vi "PECT - Scan_time gate - 2.vi"() -> ()   [LabVIEW 2012]
uses:
  <vilib>/DAQmx/read.llb/DAQmx Read (Analog 1D DBL 1Chan NSamp).vi
  <vilib>/DAQmx/read.llb/DAQmx Read (Analog Wfm 1Chan NSamp).vi
  <vilib>/DAQmx/write.llb/DAQmx Write (Analog Wfm 1Chan NSamp).vi
  <vilib>/Instr/_visa.llb/VISA Configure Serial Port (Instr).vi
  <vilib>/DAQmx/create/channels.llb/DAQmx Create Channel (AI-Voltage-Basic).vi
  <vilib>/DAQmx/configure/timing.llb/DAQmx Timing (Sample Clock).vi
  <vilib>/DAQmx/configure/task.llb/DAQmx Configure Logging (TDMS).vi
  <vilib>/DAQmx/configure/trigger.llb/DAQmx Start Trigger (Digital Edge).vi
  <vilib>/DAQmx/create/channels.llb/DAQmx Create Channel (AO-Voltage-Basic).vi
  <vilib>/DAQmx/miscellaneous.llb/DAQmx Fill In Error Info.vi
  Global_data.vi
  <vilib>/express/express analysis/Spectral/Block/exnSpectralBlock spectral measurements PSD poly.vi
  <vilib>/express/express analysis/Spectral/Block/exnSpectralBlock spectral measurements PSD WFM.vi
  <vilib>/express/express analysis/Spectral/XNode/ExpressSpectralMeasurementsBlockNode.xnode
  <resource>/objmgr/daqmx.rc
  <vilib>/measure/NI_MABase.lvlib
  <vilib>/Platform/NI_3dgraph.lvlib
  <vilib>/DAQmx/write.llb/DAQmx Write (Analog 1D Wfm NChan NSamp).vi
panel:
  in  "Open tdms":bool
  in  "Pulse generator":T1={"Waveform Type"=0, "Amplitude"=6.0, "Frequency"=1000.0} {"Frequency" format="%0.2p"; "Amplitude" format="%0.2p"; "Waveform Type" items=["Sine Wave", "Triangle Wave", "Square Wave", "Sawtooth Wave"]}
  out "Cur. X":dbl format="%#_4g"
  out "Old X":dbl
  out "Cur. Y":dbl format="%#_4g"
  out "Old.Y":dbl
  out "Compare X":dbl
  out "compareY":dbl
  out "y >= 0":bool
  out "x >= 0":bool
  out "move X":dbl
  out "move Y":dbl
  out "deltaY":dbl
  out "delta X":dbl
  in  "Move Distance":dbl=5.0
  in  "Emergency Stop":bool
  in  "Stop 3":bool
  in  "Home Y":bool
  in  "Home X":bool
  in  "Back":bool
  in  "Front":bool
  in  "Left":bool
  in  "Right":bool
  in  "Stop Scan":bool
  out "Start Pos. X":dbl=-22.5 format="%#.4f"
  out "Start. Pos.Y":dbl=18.8 format="%#.4f"
  out "열거형":T2(ring)
  out "숫자형":i32
  in  "Gate 2":dbl=50.0
  in  "Gate 1":dbl=25.0
  out "No.data":i32
  in  "Save Scan mode":bool caption="Save Process"
  in  "Plot style":i32(ring)=5 items=["cwLine"=1, "cwPoint"=2, "cwLinePoint"=3, "cwHiddenLine"=4, "cwSurface"=5, "cwSurfaceLine"=6, "cwSurfaceNormal"=7, "cwContourLine"=8, "cwSurfaceContour"=9]
  in  "Stop 4":bool
  in  "ViewMode":i32(ring) items=["cwViewXYPlane", "cwViewXZPlane", "cwViewYZPlane", "cwViewUserDefined"]
  in  "Scan":bool
  in  "Motor Trigger Source":tag="/Dev6/PFI1" caption="소스"
  in  "Open csv":bool
  in  "Tab Control 2":T3(tab)
  out "Hall sensors signal":waveform(dbl)[](graph)=[{"t0"=timestamp(3525645621.636764 s since 1904-01-01), "dt"=1.9999999999999944e-06, "Y"=array[2100 elements], "attributes"=variant("NI_ChannelName"=variant(string "Dev1/ai0"), "NI_UnitDescription"=variant(string "Volts"))}, {"t0"=timestamp(3525645621.636764 s since 1904-01-01), "dt"=1.9999999999999944e-06, "Y"=array[2100 elements], "attributes"=variant("NI_ChannelName"=variant(string "Dev1/ai0"), "NI_UnitDescription"=variant(string "Volts"))}]
  out "Feature Extraction":dbl(graph)=0.021153968958947764
  out "Waveform Graph 2":waveform(dbl)(graph)
  out "Power spectral density":cluster{"f0":dbl, "df":dbl, "magnitude":dbl[]}[](graph)=[{"f0"=0.0, "df"=238.09523809523876, "magnitude"=[-25.4340272409559, -28.495970805276507, -69.09064054555873, -79.11355871279994, -75.69366097931027, -84.18131507822396, -80.50168881348966, -82.72314293089615, -87.19630499623688, -82.83568021481967, -89.95290866002237, -85.90392585035596, -87.41269111550386, -91.40893948681482, -86.69370819914215, -93.36336146616782, -89.019380476413, -89.73232030153878, -94.58261196624535, -89.16287927388944, -94.965890302584, -91.86846413178648, -91.95327957161693, -97.62687167891286, -91.59993648735762, -97.30685711015555, -93.8350762480425, -93.27921214218685, -99.59438563802183, -93.1824258709588, -98.3113125531512, -95.45425138584356, -94.39327135467576, -100.65352961491782, -94.55889081970952, -99.40788907105079, -97.93617495318924, -96.19517579047603, -103.97036797797732, -96.40295202889732, -99.7036956909043, -99.48760137175819, -97.46192979187015, -106.29271483151813, -97.51447379981207, -99.86179280251669, -100.43811038443037, -97.59011642740829, -105.58363666166275, -99.01126121197593, -101.01575323613292, -101.90167607549864, -98.61952569586691, -106.73670466995647, -99.29976101634999, -101.54959604687718, -105.17330050767885, -100.09392305285375, -109.78264848704497, -100.98914236173123, -101.81665207962125, -105.42358374403365, -99.82880728595141, -107.07330885402075, -101.07712607444097, -101.03780825357597, -107.32811151840846, -101.221643458408, -105.63776326231454, -101.8420593566944, -101.80081629073969, -107.47915505307212, -101.12986632760553, -106.84901404755908, -102.73715610491038, -101.51552854007832, -107.28771371003282, -101.3928633472346, -107.44515355816633, -104.89304864643535, -103.1455098860718, -110.19910428997925, -102.73063833081197, -107.57101838377707, -104.90574568581201, -103.72599931018533, -109.97178587260123, -103.24611921258705, -108.36098023558972, -106.6408311450923, -104.73569536588386, -116.21683530762306, -105.02627439976544, -107.15856030450797, -109.81191038702062, -105.53476822084077, -119.10077766590356, -105.31867536160968, -106.9718410299748, -108.34458911268797, -104.70307996109247, -114.76704583683203, -106.29948298493936, -108.55077108437321, -112.16618350190343, -105.98453547558171, -114.68576835450673, -107.50968901677987, -107.89174277914348, -111.59875709602721, -106.69368240333122, -114.93273233954758, -105.23904516482949, -106.00272331017348, -110.36103151258544, -104.93177986717492, -110.8835476773746, -106.69346348818806, -106.66103973993782, -119.11729839814336, -108.06338160849775, -114.5879267769655, -108.59816838472844, -107.53189260743514, -114.07390818184973, -106.70996756049796, -113.27381274118753, -109.50270539577696, -107.37282420343303, -113.4779718725949, -106.04267666963091, -111.30294425571472, -112.46717993668915, -109.13164915488709, -116.65287200885172, -107.03002573045511, -110.21479040603631, -112.476075561056, -106.97710947409149, -119.42145279296255, -108.3200486628316, -110.46641858585929, -117.16650627564961, -109.73297826697552, -120.31689830731365, -107.19513745371916, -110.66663569403087, -113.30365980039964, -110.01971553524372, -123.68660617105166, -110.8171755739396, -111.11382172813546, -117.76239209582961, -109.49899370205401, -115.22252846498625, -111.1932077339224, -112.38235939086871, -118.22207022901702, -110.6546796895719, -116.97450780644367, -110.82401674194465, -111.96705198878843, -118.28092956599232, -110.5621503678909, -121.25720613496851, -111.98371482341479, -113.27928013246557, -111.96833712758355, -108.56859286664552, -120.32790468431601, -110.82699792221703, -110.79062667340345, -122.65756767769517, -110.48843456045427, -116.8782055296399, -115.43719816168479, -114.47619780315773, -121.42183196132746, -111.60631415727042, -120.68077308056417, -109.35478690141552, -109.03210709352732, -120.6260555904793, -109.47936424950136, -113.33719701518146, -112.88325992990137, -110.99901978536154, -123.19636626521421, -109.09861317900774, -113.33125158106256, -115.35673297389727, -112.77249677632989, -124.61163141716472, -114.68140920359865, -121.89642913325117, -115.47413298424323, -112.82196063671608, -127.87542521315149, -111.54178118788309, -113.6448752704395, -120.76569423868874, -112.98651214877823, -123.18868565400437, -115.41399838634062, -115.46853076016815, -116.40989072804102, -110.69611347288615, -132.23164080331392, -114.76376391429793, -121.7246597336247, -117.46893009589195, -114.01899156779395, -125.22079066032327, -114.59524199183258, -114.50034890537415, -122.9532092227648, -113.72727798159212, -125.65163915514907, -113.4793801211504, -110.4090756414644, -125.63592649005872, -114.22938378193007, -116.74947251106808, -121.60535557984142, -116.79385283402802, -122.44667696630361, -113.43873413563811, -123.28159708694415, -113.92892974938164, -114.01193823589753, -121.62751955742443, -118.76839573694522, -125.52998605097204, -115.19609643487229, -117.49409595176479, -117.08423885198002, -119.48314867245172, -125.01675515413412, -117.92668164142911, -115.55962389856793, -125.63488616674975, -119.11862859365166, -114.78860770332909, -117.18339781294443, -111.18063004722558, -118.31775966044624, -111.6867367949252, -114.57226159377, -119.36541212960576, -113.90245139442648, -132.46343443313128, -120.1282759002165, -121.05279009698619, -118.9115822659523, -121.23280439248342, -116.31914159559688, -127.38829313950257, -117.34673005740623, -115.95249861902771, -114.9301657394146, -123.22361802797445, -110.83274939062106, -116.16624248562111, -116.76753364192771, -113.94454545069023, -122.95736945775944, -118.66755800656253, -129.1462641201204, -116.6351050110328, -117.22529407303742, -123.80212197360244, -115.89792176423389, -114.25823938606595, -125.60467961977515, -114.59958849364433, -121.70071005514421, -118.25968972451209, -114.69929400946009, -123.88209034116528, -115.03869272537257, -117.52034211782204, -115.27990843516797, -117.85366603932033, -125.16865559622727, -118.21960424638507, -119.69008755413566, -117.24640963460672, -114.32867295013791, -119.1576982419508, -122.85495988425586, -116.3373010103401, -114.53730203699834, -115.67017599990201, -127.144321037601, -115.73849102686786, -117.7626163106355, -119.7346592991025, -117.41317517684553, -125.0417974461613, -114.5488949833583, -116.59812516173781, -119.91064563147799, -115.27933218667663, -122.09990513751134, -120.95678574143693, -123.25641714743752, -112.5173710452192, -113.53735878806998, -129.23914933506734, -116.27157269711533, -148.4020512032711, -118.84888216023774, -123.82550527215588, -116.87770979616658, -111.32191810025745, -124.32675905891588, -114.37182733794062, -121.10713785851372, -122.59698730059695, -116.38346694563282, -121.69144349152856, -119.00883142493832, -110.81886738196273, -120.7909830607913, -115.01780448665316, -114.52055121633796, -132.6824191654361, -116.330695115645, -126.4664151018508, -118.32717907779282, -118.7288071595281, -120.42749846140066, -112.53185615773879, -124.26026008984286, -114.24089252048742, -120.00368190003405, -114.71738500842926, -112.92262025927133, -129.21127897188563, -113.5947811765517, -117.80802009651353, -117.0133790103226, -112.19210322760304, -118.17549968071762, -119.3256187825503, -118.84981507334446, -121.39118969751144, -114.64543555194373, -119.84814933224528, -114.09123407848944, -116.22899352170892, -116.41650104077173, -113.70057202673476, -124.52773908304957, -114.87372641784933, -116.11651108221098, -121.68680962246994, -115.78306007961302, -122.22621008657796, -118.81157995182392, -113.9402115821658, -132.636729517989, -114.49554876936634, -119.50980190398928, -123.27410972236837, -118.52851881066383, -122.25212982572599, -117.13947036230024, -120.85005588797962, -118.41526503460501, -117.61788553858068, -126.3872056783977, -114.98198608543298, -119.7789938911847, -120.84873579392627, -114.38831474301695, -153.35954756825245, -113.19505610638078, -114.17454820985151, -127.41069917723112, -114.92677241657191, -125.49053973810628, -113.36382196587914, -119.96785250843519, -122.47388530423243, -116.38671253508838, -120.0905790211523, -119.83326265062107, -117.88168146696918, -122.3132169880757, -115.87324909105399, -125.92003267803432, -113.96860176867415, -114.49156118371398, -127.52634390035722, -115.05967156528004, -126.82020221981517, -117.93643187259194, -116.51163213641807, -119.47551219110167, -119.55225172256931, -116.9512257852571, -122.23153124485954, -120.8368476753637, -121.48473913072222, -115.83122660909913, -135.74260014140523, -116.58358375805423, -118.15236945484727, -119.06674062398864, -115.7844834762477, -125.06111738611818, -114.7801535050972, -115.2696605691888, -123.98656374010793, -119.29025555731172, -118.29146803784099, -119.55696172158135, -118.06884171238352, -127.81587648134607, -120.41730580797976, -123.49626136731604, -112.2147141798107, -116.22555232584983, -132.79419178871254, -119.66964883124663, -117.20946469243259, -118.20939292735417, -115.6951914646649, -129.64892855822356, -114.27056999288617, -120.31005512957381, -117.41846777372632, -115.50158386260813, -124.69777160737624, -115.2892897247205, -123.61522771666871, -113.75248734362687, -113.22999749252833, -129.3490509395313, -116.88137735661701, -116.94110280242681, -119.50244079984806, -119.30521139999144, -128.17199984115797, -118.06736594940236, -116.05331575995922, -121.29670750650897, -116.1140297602044, -125.090619084802, -121.41807296062154, -120.01332757902264, -120.54914530643151, -116.49738633175463, -122.32551291835904, -118.3190808346865, -118.92638453656723, -122.48819531011718, -117.01021725424317, -120.98896352560598, -117.23831688685218, -121.27915259197124, -121.20017251921661, -117.6155648860373, -120.91300272912063, -117.94438460863424, -115.94437430101533, -123.35904829443987, -117.74011174503076, -121.54935745388448, -120.82564553545025, -121.98951430455743, -120.24858103448778, -116.44403527138395, -112.79571494351876, -112.42801913096545, -110.1697573019791, -115.34500457736401, -119.81921052956707, -129.82600951154313, -115.5862301263047, -112.59292882433087, -120.79009137478283, -131.32849293387295, -113.61194478398238, -123.48568856527031, -119.17507777781304, -123.09261867490484, -116.97755217417308, -123.94453461434183, -116.58080525616379, -119.64289646280756, -122.90202645580743, -126.66219093058154, -121.95048829056148, -115.72578023509817, -116.70117814464484, -121.91050280869723, -118.25299095698178, -116.45905559047064, -132.57794493731578, -121.65327820443292, -120.9816664775787, -117.17270262269045, -120.27433984830965, -125.89418976028173, -119.09563505847817, -126.9693215534833, -113.17465524665704, -118.98702092883116, -119.83822568580342, -120.45832738089722, -120.67735960513633, -127.38676010839353, -127.65777338183055, -118.37446329057411, -115.61355494839711, -119.94568688114103, -116.06619937633681, -126.348857777089, -118.92850079147068, -119.5416617639739, -132.47075644221843, -118.08809356028496, -123.16186463092723, -121.51579486791232, -122.88983670053283, -129.5195538417256, -120.4730389608841, -132.16486858341602, -122.34690358436781, -120.71922104337597, -114.29260860841114, -117.67902631803368, -124.7040155514909, -123.51274592117205, -120.02297921674332, -136.54655493811157, -120.45629227407751, -119.06410204276258, -127.91681714792554, -122.82090055753153, -125.16838176650813, -121.79565386970478, -119.79607311590995, -126.54861375039647, -121.59135878113302, -132.8348640697562, -118.1305434733294, -120.46070148841905, -122.69571910896963, -117.6534954653865, -124.15742546824006, -120.73646926947502, -124.82696993800742, -124.513836786494, -123.15395713389651, -124.62395468806395, -117.21365768658171, -119.32635871968456, -121.48532284413152, -119.38242892643675, -126.25575652510352, -123.27133124029851, -117.58533922728374, -118.17710108929799, -114.99496360200965, -117.77133194647278, -111.34898201101595, -111.50817058307922, -119.0703124690998, -127.70676079885351, -121.8704969141074, -125.93154214283446, -118.65628450081473, -122.47918878348962, -117.9651589546518, -126.13560583004508, -122.42294805637847, -133.924453763793, -117.2082573038767, -117.6525335446734, -122.92077297426977, -122.04624645756786, -116.43289028226238, -117.93180959338378, -129.02356734231915, -117.95493621286326, -120.7555929766252, -120.76782849311112, -123.06287498470708, -117.83798593857965, -123.43423215434719, -120.15190119516652, -120.48240443128407, -143.29738987393452, -123.46572247444769, -120.89055325172792, -125.66715973809033, -118.26887578998644, -117.01836200028421, -121.33021830755509, -119.68846363313813, -122.60689066103069, -116.26858138914181, -119.59360791972998, -122.94866175463353, -114.174409515556, -118.00516930888391, -121.56978543579633, -135.87799017759036, -117.50816594504829, -122.82539428457626, -123.82103443155845, -124.77975840345442, -121.13340798086698, -120.93607435603558, -133.15787160745222, -120.70545628137863, -125.02155972441679, -122.04666465472178, -118.01234649746348, -127.88767491042842, -119.02096620167217, -120.16031065152875, -122.25406107859625, -121.72733059051095, -120.61357375519918, -118.63962847172827, -134.3857741605498, -116.3600853185034, -117.26695700691671, -119.9176982185873, -113.45576465218444, -126.69779573632724, -114.39554522802246, -116.8457146515868, -116.34219889483086, -119.30011291548334, -120.01163291843496, -114.29497178248809, -127.65687642749229, -119.58556923753022, -129.8593054181261, -122.2353645100479, -120.79536520223796, -119.83284028355028, -117.7991246185715, -128.390292904734, -119.78079925213122, -125.478913448993, -113.89747777944768, -112.66620124153357, -124.3475049842711, -120.85847303094337, -132.91807981902295, -119.523494985723, -116.65149909866443, -119.73287290436721, -127.63237851524192, -127.23413304048789, -120.87585453904362, -121.08540368080186, -134.91071939669257, -117.75375801669338, -117.2683014590723, -120.9739099492833, -118.23809733632451, -120.94065804928206, -123.88077510875804, -118.13812819300607, -122.60294123365466, -126.97075898006995, -120.18754789731035, -124.71238663441227, -120.55456557278582, -130.94599087480253, -111.18288669417035, -112.27708791831247, -126.0512034600378, -117.41881712783596, -128.20553880273903, -117.29482600885808, -118.2045526390752, -127.81966672699878, -117.03716165902529, -115.46711739757512, -117.15363929234843, -121.87599671671335, -121.19736800869221, -126.5301786755875, -131.20754947382918, -124.40138004810741, -129.0562496906515, -121.06816554587536, -121.01023627802867, -138.6137911215848, -120.12495002524031, -121.38510517514229, -122.79804220535513, -116.97501378195477, -118.82011581137473, -114.0229185604644, -119.54287501990726, -114.64474566771625, -117.76935669872461, -123.81082574158907, -118.51678358865587, -128.9664755188374, -123.45357998434133, -122.74888841574231, -120.74640581234044, -126.956344345126, -119.95682140104577, -118.8873101779055, -124.41062359284174, -128.97304498664363, -123.86287113204068, -127.30257087528216, -120.61364220528216, -114.45119129304715, -119.68384044686806, -131.29639185291157, -122.31250766293485, -119.57420865241102, -124.74014026002448, -124.87593035709094, -118.4566565612952, -123.76236085976001, -120.84780538841838, -117.68987599773281, -135.06195695255914, -122.56143585795171, -129.04610316842883, -118.32313199570537, -117.77093802786419, -124.46572845786741, -129.1123298336903, -120.88470269965448, -116.69988985752187, -116.84054667499878, -133.76883696987278, -122.32434984927302, -124.98940594457933, -122.56515592789917, -118.31562562243366, -133.97049179545627, -122.33220627999802, -131.16753675316977, -124.69828063969263, -116.37621154460467, -126.1833423168025, -129.62937634161355, -118.46241371150788, -117.52851478852457, -125.32425037236442, -119.0327364293772, -124.2861355894013, -123.24573502278234, -125.52155812053758, -113.75743410709823, -114.79513162658353, -128.58142362588052, -122.48277095196701, -118.94747544412269, -123.86988127835491, -124.78140456983323, -121.53998481875398, -116.01432822539552, -119.20174681160661, -122.75167725800814, -120.58657749420254, -118.51141061842183, -119.24457006171983, -131.43641234223372, -116.00759139055087, -121.24442216102587, -123.29371279953725, -117.608355420454, -116.33684374617326, -118.06291688281922, -121.88761866022774, -121.54820313120047, -119.5051369873635, -126.56611158390913, -118.84012713615805, -121.09285296522563, -124.67955377692547, -147.31451139022337, -116.80660421066897, -114.8367853755961, -120.41026468628925, -123.65666101895222, -119.64837119787269, -116.77480172559095, -116.54263359173909, -124.75286620868079, -117.33721912698883, -116.51795620907136, -118.50086748176733, -128.10381328920522, -122.78098994574157, -120.24716756092855, -119.52743204722819, -115.00407387659232, -108.2853711552629, -108.61086943894702, -119.6228894146785, -124.11132022420912, -125.6202218409766, -123.1749360787656, -118.1971196161698, -123.95075368058998, -121.72140109898365, -123.27106899042522, -123.73035629887062, -121.24369679109273, -121.07381526465288, -113.13965659723667, -118.330755475899, -118.40249076804484, -111.59630598649044, -116.1569506845575, -125.67326089915758, -125.85723567111906, -119.24293277595024, -117.87067617433537, -120.70936924059559, -131.8090588468898, -132.98711569625004, -123.63274249467587, -122.75476917502559, -126.12873814250243, -120.53144270605179, -129.07030822919336, -122.7889410422919, -124.35405971166259, -119.63968579420454, -139.0154441054289, -129.47962001806934, -121.86548015410847, -128.6818469257012, -121.40195873232601, -138.64231053781285, -124.22025721762265, -124.06073958736941, -126.71929802352521, -131.7498459276443, -120.68144109742178, -122.6325588818875, -126.80796617875095, -124.92487955227033, -136.94498040498806, -124.26704334219014, -123.21376211221711, -140.25352033075964, -129.53222319772195, -122.58541579060463, -122.1996729592375, -125.66642108013673, -125.66310429236694, -120.09682773706965, -125.27326633941439, -121.55721878725502, -121.22507119941083, -121.53716878624485, -136.20685498111987, -128.15260146013156, -120.03473972471616, -124.60755958763912, -124.73082500077143, -123.93425949983688, -131.04483249265184, -121.7957035014449, -127.09321441816094, -133.6144579272493, -124.69014595896968, -130.4902091211609, -121.18031440773905, -128.00033943961677, -125.88991118115149, -118.865310745079, -123.69668867733147, -117.98756965862728, -114.40013091842827, -118.28685032521078, -122.23464196869948, -124.8440422629961, -129.66281606870848, -119.440534215621, -124.54391783563877, -124.93447967158188, -121.7258558761523, -122.28817885403082, -127.06889620458577, -128.92172974939206, -120.62932166634072, -126.06847321900452, -123.31471168429935, -121.80350826545656, -129.2574604322076, -125.67225933193998, -125.7801671825605, -129.53804733161627, -119.56756644124712, -128.82490314699373, -124.7689736295626, -120.50019729114693, -124.50603158563972, -122.8120627011088, -125.60528875555717, -123.8817354922713, -124.05570537836674, -120.94568834491936, -118.06056028605255, -124.24390361274648, -125.5716703018188, -127.71949519914061, -130.7001652968252, -126.27701412017494, -133.76810134709916, -128.4738939614179, -120.302550881701, -118.91298143662928, -124.9077318110765, -127.16253699189492, -118.11405934812818, -117.52028071290711, -140.95620572748925, -123.61977932545628, -131.0334379970501, -125.88948384968432, -127.81552331993379, -121.92316280719056, -119.05911238768732, -126.83773251459189, -123.52627415002164, -120.8779561023192, -123.66683567603742, -131.64300993967345, -123.62895847772963, -116.89792951363142, -120.1068259250195, -117.92484706459337, -115.58208487778379, -120.76803581628594, -123.95408562090736, -122.79456549632754, -134.5305398779298, -123.57040300991032, -128.40634159414552, -123.70102187824159, -118.24970739397313, -119.66483900349026, -127.78024313111393, -120.3547204111785, -125.49305364308705, -119.49505591004302, -120.50920386196539, -119.03509516851003, -114.24667300009652, -121.60538636584391, -119.95304417598024, -122.24585853682832, -128.63653016912684, -116.04810628805795, -121.94159862131235, -122.59928204398939, -121.4532410501923, -128.6511474663462, -130.83715595958148, -121.71998300574741, -116.91426629511156, -113.587592058512, -115.59736707638731, -124.65300822631244, -133.32538684258748, -124.02289142873636, -121.54278890993639, -119.02596809402394, -108.90572887117857, -112.14974069608851, -129.21149299565423, -118.82148342951197, -116.65510894288538, -118.39609618084175, -116.53502642884725, -122.47549439965209, -122.23125657046063, -123.68081343116663, -120.67915071600007, -123.6899360128769, -118.56721985209728, -118.36641581191942, -126.96724630704657, -119.36877661672403, -123.07698921198843, -117.80772421906035, -122.82545076270567, -118.82755071380888, -117.21030132539394, -129.760567864525, -118.0816708063509, -125.80573274113647, -121.18434666182338, -121.80987210832065, -130.99259828357094, -125.47223579895922, -123.86818606677002, -118.7118158196511, -119.27778317338742, -127.27333258839096, -119.90672352079164, -140.78772370844268, -118.08251080057329, -119.86636232122572, -118.69482489738232, -119.19106512767372, -123.70988914879189, -121.92566832147995, -123.41378261726373, -120.1715186070818, -117.9079629421116, -117.41960207545632, -123.72833996166874, -127.24377206607298, -124.99098647980887, -129.48803701799955, -129.92351350561592, -120.79284154834647, -119.29601975194524, -136.17244775530037, -126.73975437546255, -128.84068276143336, -125.66374985701982, -136.69026010435715, -125.44409235146617, -119.28138070315057, -118.65017329869724, -118.02521532826772, -122.23736063759657, -121.27846943548622, -116.69850478126861, -119.7711336696722, -123.70776561180185, -118.43344549561263, -123.92390877157247, -117.19637143066551, -117.64112988205311, -127.78399195238529]}, ...(2 in all)]
  in  "3D Surface":refnum<k7>(container)
  out "Record path":path caption="selected path"
  out "Feature Extraction 2":dbl(graph)=0.021153968958947764
  in  "Tab Control":T4(tab)
  in  "Step X":dbl=0.1
  out "Move X":bool
  in  "Direction (+)":bool=TRUE
  in  "Step Y":dbl=0.1
  in  "Y-length":dbl=10.0
  in  "X-length":dbl=5.0
  in  "Save Speed":bool
  in  "Cur. Pos Y":dbl=18.8 format="%#.4f"
  in  "Cur. Pos X":dbl=-22.5 format="%#.4f"
  in  "Travel per Pulse (mm)":dbl=0.002
  in  "2 Rate":dbl=0.2
  in  "1 Rate":dbl=0.2
  in  "2 Min":dbl=1.0
  in  "1  Max":dbl=8.0
  in  "2 Max":dbl=8.0
  in  "1 Min":dbl=1.0
  in  "Parity":u16(ring) items=["None", "Odd", "Even", "Mark", "Space"]
  in  "stop bits":u16(ring)=10 items=["1.0"=10, "1.5"=15, "2.0"=20]
  in  "Data bits":u16=8 min=5 max=8 step=1
  in  "Baud Rate":u32=9600
  in  "COM Port":refnum<visa-resource-name>="COM12"
  out "No. X":i32
  out "No. Y":i32
  out "Sample per Channel AI":dbl
  out "Sample per Channel AO":dbl
  in  "Pulser Cycles":i32=10
  in  "Logging Mode":i32(ring)=10231 items=["Off"=10231, "Log and Read"=15842]
  out "Actual Sample Rate":dbl=500000.0 format="%0.2f"
  in  "Physical Channel":tag="Dev6/ai0"
  in  "Min Voltage":dbl=-10.0
  in  "Max Voltage":dbl=10.0
  in  "Terminal Configuration":i32(ring)=10083 items=["default"=-1, "RSE"=10083, "NRSE"=10078, "Differential"=10106, "Pseudodifferential"=12529]
  in  "Sample Clock Source 2":tag="OnboardClock"
  in  "Sample Rate":dbl=500000.0
  in  "TDMS File Path":path
  out "Actual Sample Rate 2":dbl=800000.0 format="%0.2f"
  in  "Physical Channel(s)":tag="Dev6/ao1"
  in  "Min Voltage 2":dbl=-10.0
  in  "Max Voltage 2":dbl=10.0
  in  "Sample Clock Source":tag="OnboardClock"
  in  "Sample Rate 2":dbl=800000.0
  in  "Offset":bool
  in  "2 Plots":bool
  in  "Edge":i32(ring)=10280 items=["Rising"=10280, "Falling"=10171]
  in  "Pulser Trigger Source":tag="/Dev6/PFI0"
  in  "Duty cycle %":dbl=50.0 format="%#.2f"
  # "Pulse Shape"
  # "Trigger Settings"
  # "Data Processing"
  # "Time gate = %T"
  # "Pulse"
  # "Hall Sensors Signal"
  # "Feature Extraction"
  # "Power Spectal Density"
  # "COM  Setting"
  # "Speed  Setting"
  # "Scan  Setting"
  # "Pulse  Channel"
  # "Pulse  Timming"
  # "Sensor  Channel"
  # "DAQ Timming"
  # "Logging Settings"
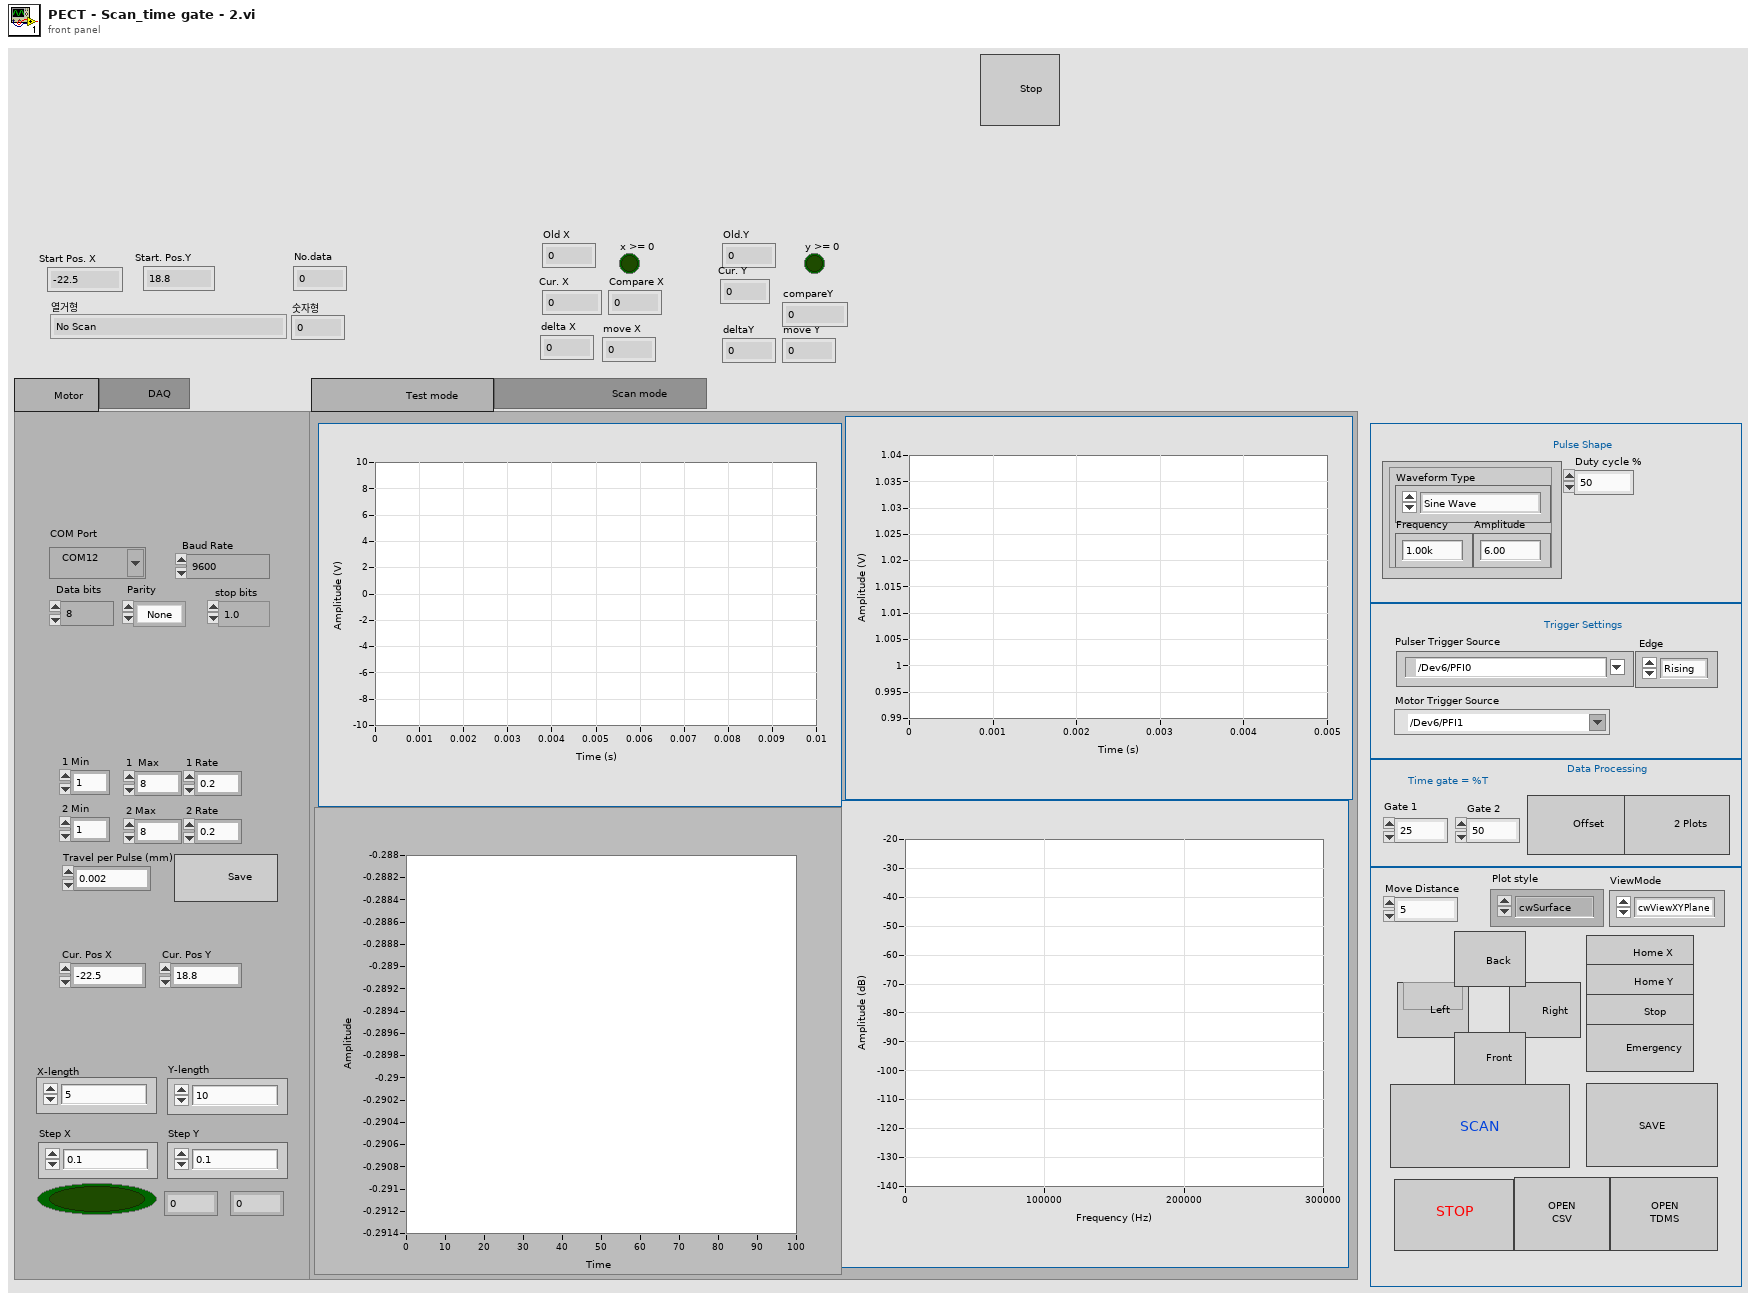
[diagram p1: front panel]
types:
  T1 = cluster{"Waveform Type":u16, "Amplitude":dbl, "Frequency":dbl}
  T2 = enum16{"No Scan", "Move X", "Wait to destination X", "Move Y", "Wait to destinatioin Y"}
  T3 = enum32{"                    Test mode                   ", "                          Scan mode                      "}
  T4 = enum32{"        Motor      ", "          DAQ        "}
  T5 = enum16{"open", "open or create", "create or replace", "create", "open (read-only)"}
  T6 = cluster{"averaging mode":u16, "weighting mode":u16, "number of averages":u32}
  T7 = cluster{"dB On (F)":bool, "unwrap phase (F)":bool, "convert to degree (F)":bool}
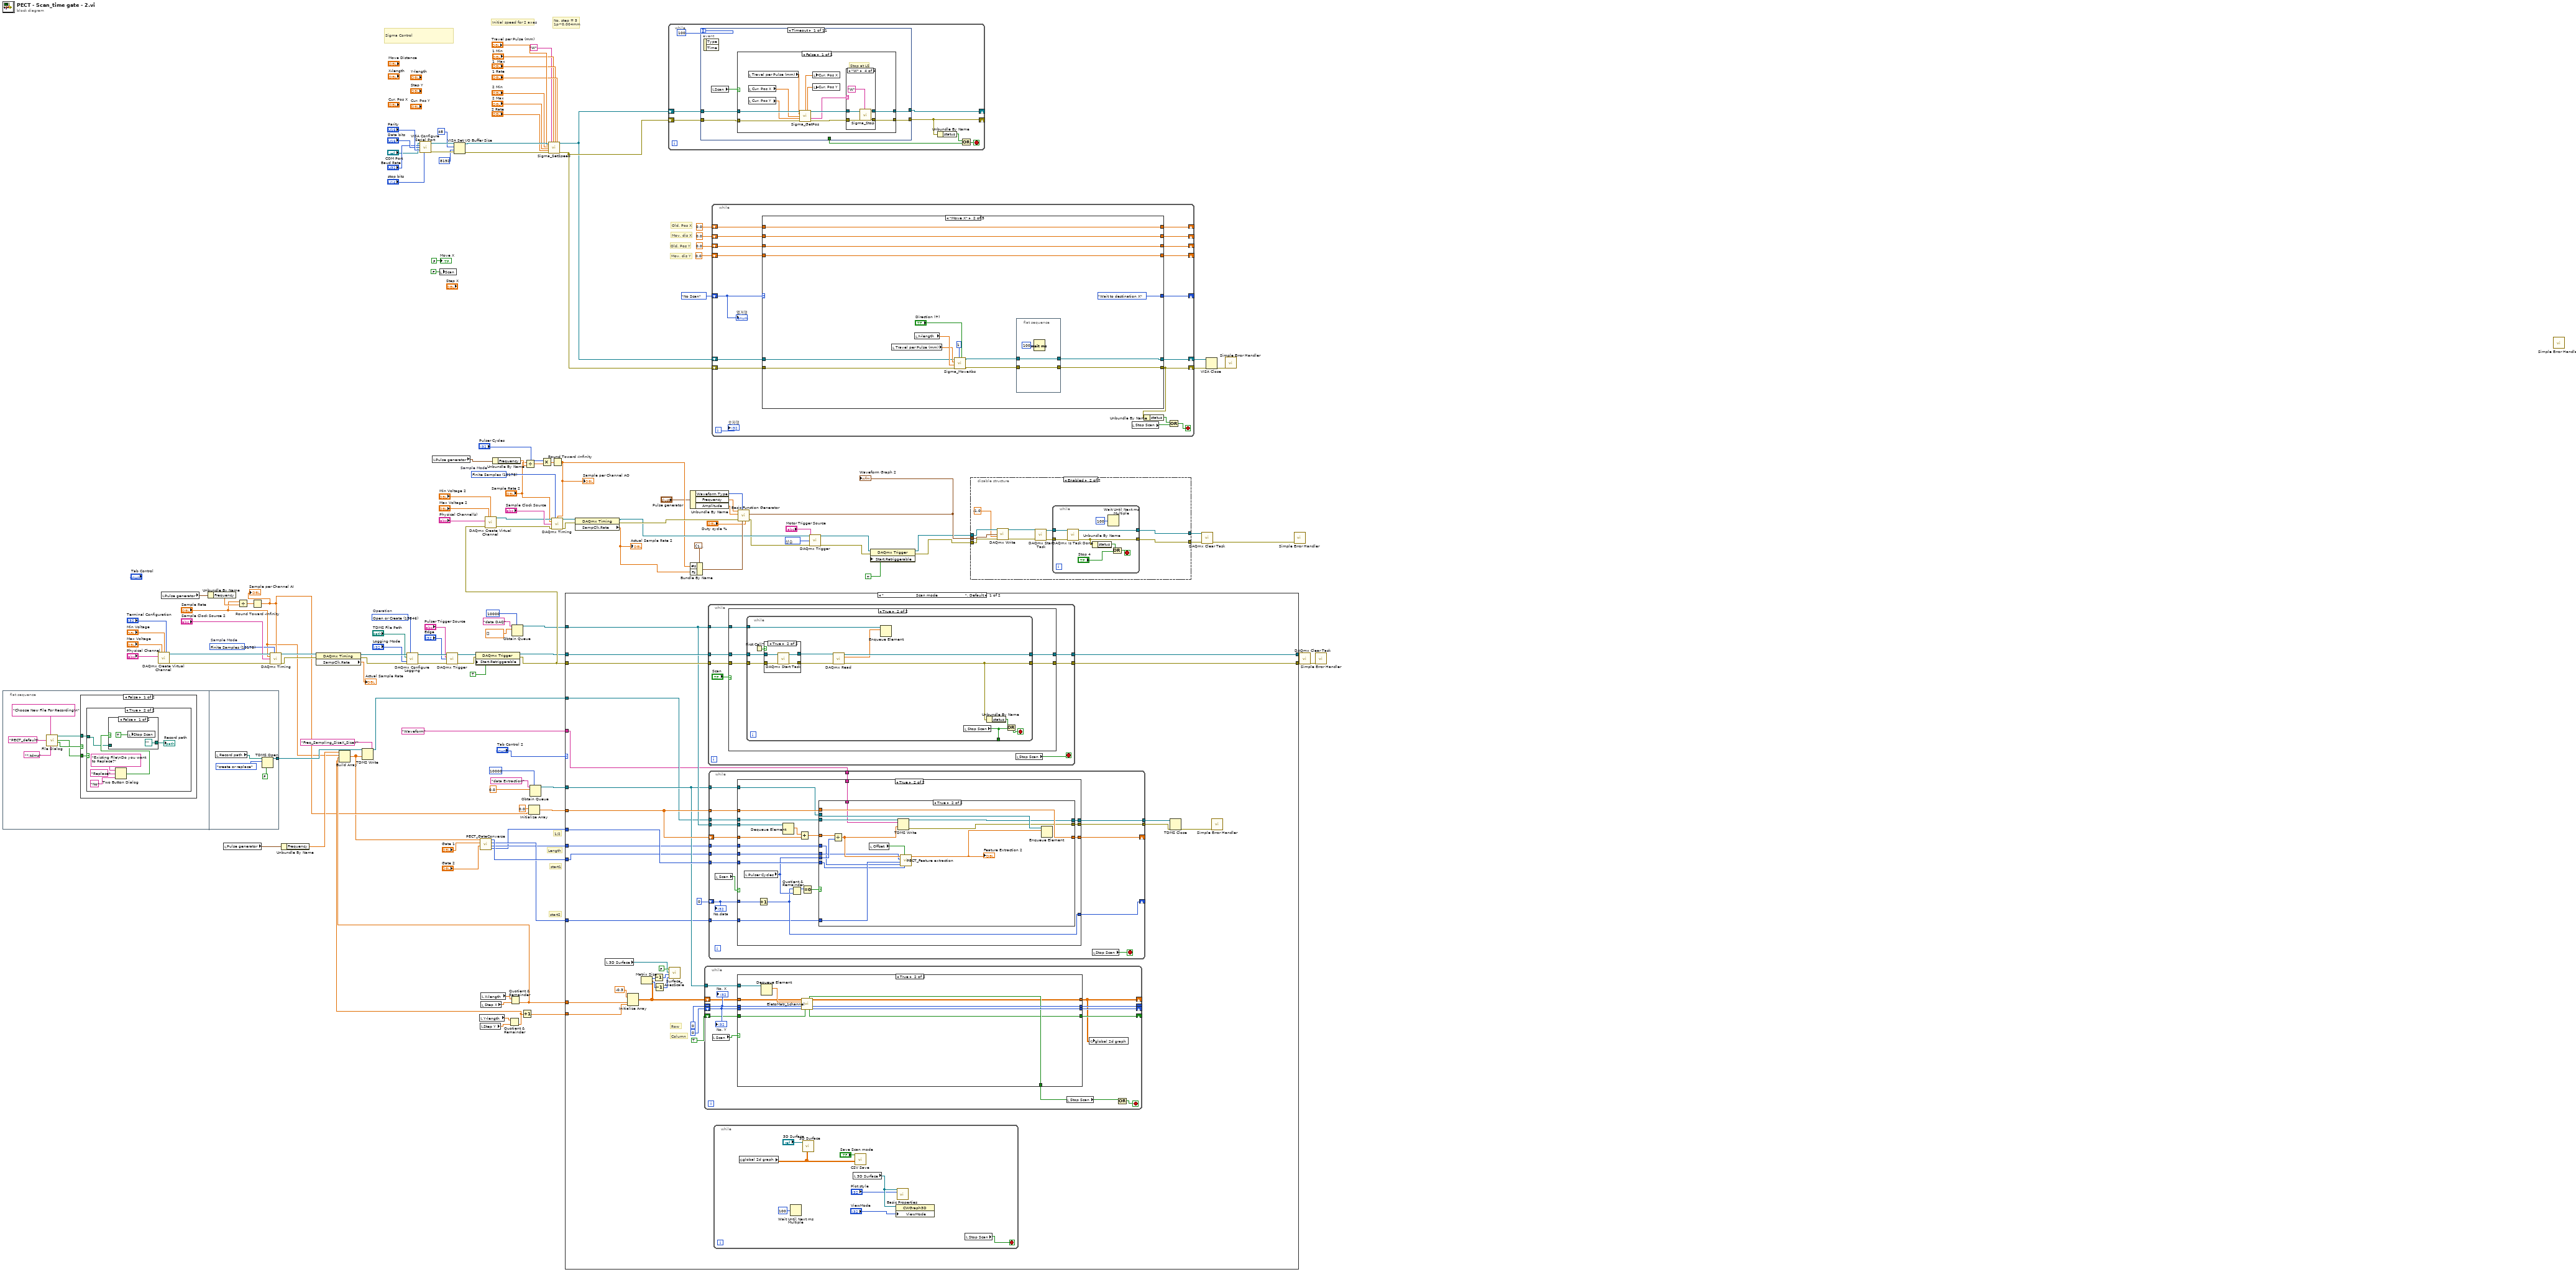
[diagram p0: block diagram]
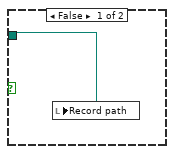
[diagram p2: hidden frame]
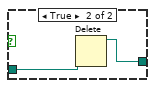
[diagram p3: hidden frame]
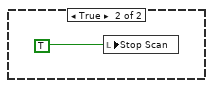
[diagram p4: hidden frame]
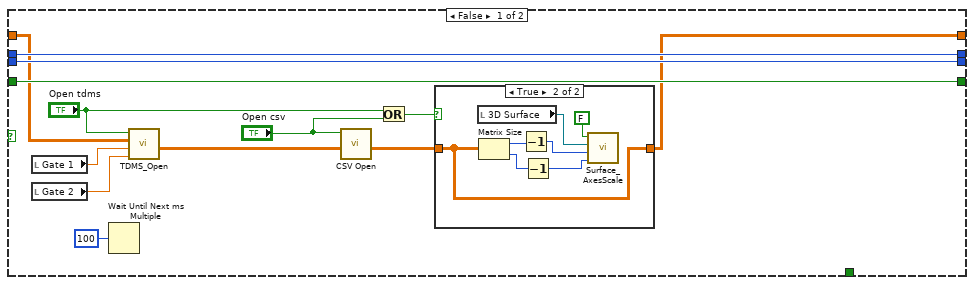
[diagram p5: hidden frame]
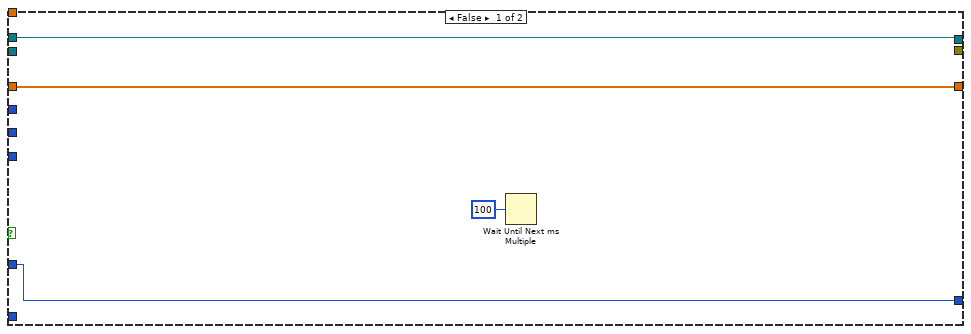
[diagram p9: hidden frame]
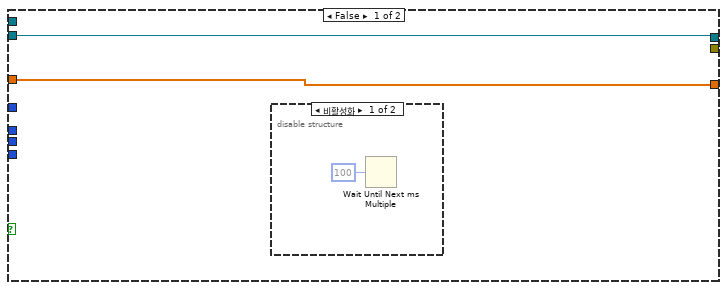
[diagram p10: hidden frame]
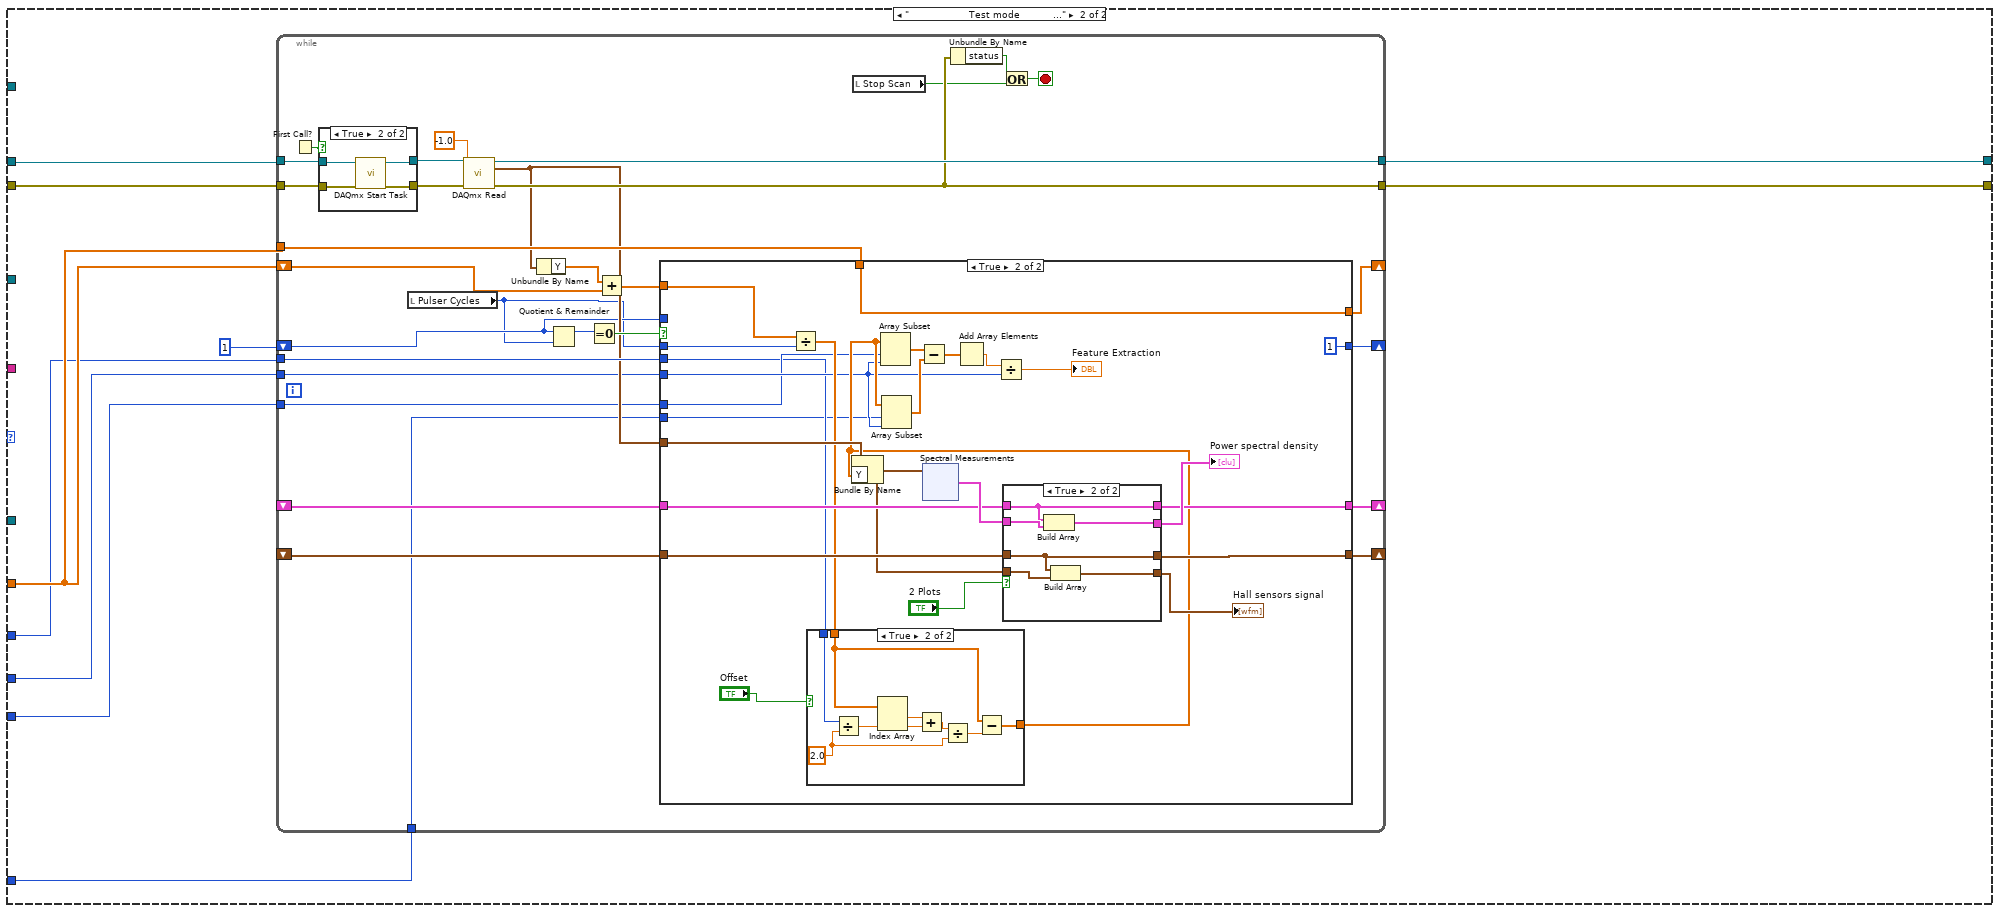
[diagram p12: hidden frame]
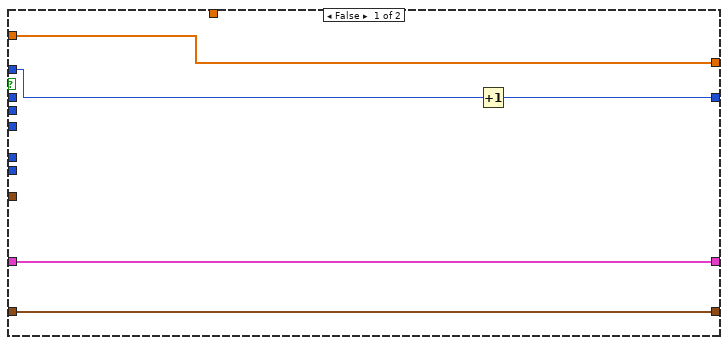
[diagram p14: hidden frame]
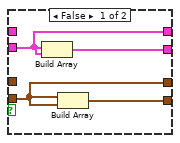
[diagram p16: hidden frame]
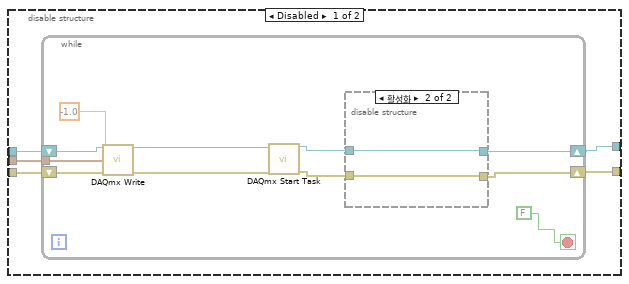
[diagram p17: hidden frame]
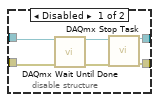
[diagram p18: hidden frame]
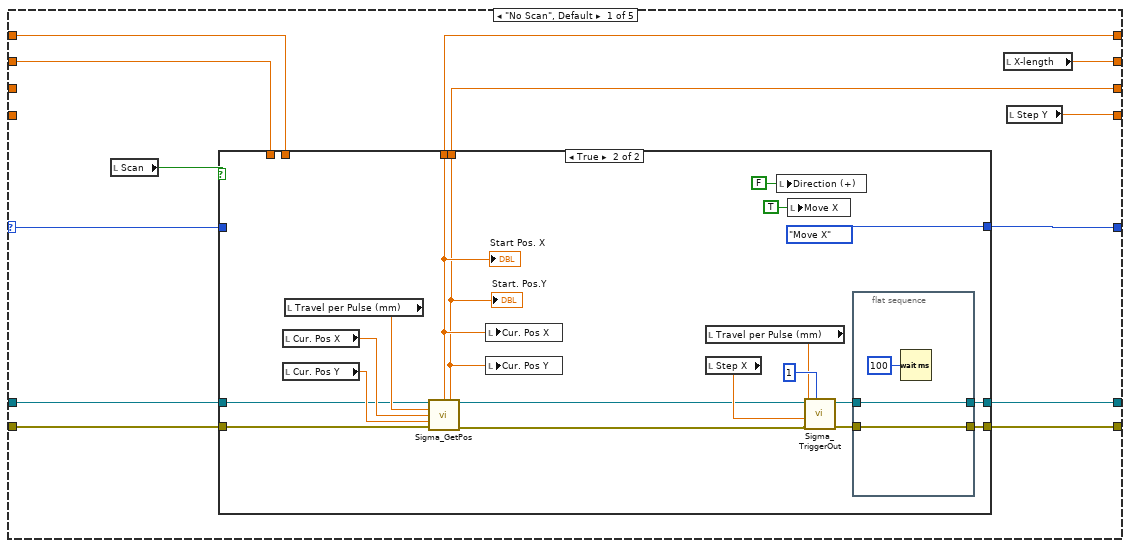
[diagram p19: hidden frame]
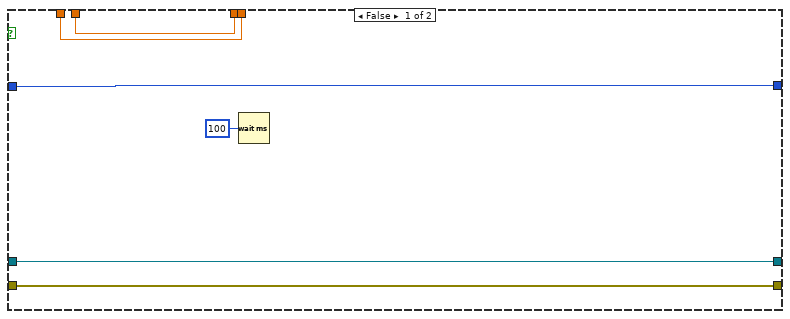
[diagram p20: hidden frame]
diagram:
  w51 = 10178 items=["Finite Samples"=10178, "Continuous Samples"=10123, "Hardware Timed Single Point"=12522]  # Sample Mode
  w66 = 15846 items=["Open"=10437, "Open or Create"=15846, "Create or Replace"=15847, "Create"=15848]  # Operation
  w89 = 10280 items=["상승"=10280, "하강"=10171] ("edge")
  w103 = 10178 items=["Finite Samples"=10178, "Continuous Samples"=10123, "Hardware Timed Single Point"=12522]  # Sample Mode
  # "1/2"
  # "start1"
  # "start2"
  # "Length"
  # "Mov. dis Y"
  # "Old. Pos Y"
  # "Mov. dis X"
  # "Old. Pos X"
  # "No. step = 5\n1p~0.004mm"
  # "Initial speed for 2 axes"
  # "Sigma Control"
  n1 = flat-sequence {
    tunnel: [w155] -> w27
    frame #0 {
      n2 = call "File Dialog"("prompt"="Choose New File For Recording\n" ("button label"), "default name"="PECT_default", "pattern (all files)"="*.tdms") -> ("selected path"=w139:path, "exists"=w134:bool, "cancelled"=w135:bool)  [unwired: 9 in, 1 out]
      n3 = case shown="False" w135 {
        tunnel: w139 -> [w140 _]
        tunnel: w134 -> [w141 _]
        frame False {
          n4 = case shown="True" w141 {
            tunnel: w140 -> [w142 w143]
            frame False {
              n5 = local write "Record path"(w142) -> ()
            }
            frame True {
              n6 = Two Button Dialog(message="Existing File\nDo you want to Replace?", 1:"No" ("F button name (\"Cancel\")"), 2:"Replace" ("T button name (\"OK\")")) -> (T button?=w144:bool)
              n7 = case shown="False" w144 {
                tunnel: w143 -> [_ w152]
                tunnel: [path "" ("deleted path") w151] -> w145
                frame False {
                  n8 = local write "Stop Scan"(TRUE ("Exit")) -> ()
                }
                frame True {
                  n9 = Delete(path (use dialog)=w152) -> (deleted path=w151:path)  [unwired: 4 in, 2 out]
                }
              }
              "Record path" <- w145
            }
          }
        }
        frame True {
          n10 = local write "Stop Scan"(TRUE ("Exit")) -> ()
        }
      }
    }
    frame #1 {
      n11 = local read "Record path"() -> (w154:path)
      n12 = TDMS Open(6:FALSE ("disable buffering (T)"), 10:T5."create or replace" ("operation"), 11:w154) -> (3:w155:refnum<k34>)  [unwired: 3 in, 1 out]
    }
  }
  n13 = call-poly <vilib>:"DAQmx Create Virtual Channel.vi"("maximum value"="Max Voltage", "minimum value"="Min Voltage", "input terminal configuration"="Terminal Configuration", "physical channels"="Physical Channel") -> ("task out"=w69:refnum<k21>, "error out"=w70:errorcluster)  [unwired: 10 in]
  n14 = local read "Pulse generator"() -> (w3:T1)
  n15 = Unbundle By Name(w3) -> ("Frequency"=w31:dbl)
  n16 = local read "Pulse generator"() -> (w2:T1)
  n17 = Divide(x="Sample Rate", y=w31) -> (x/y=w30:dbl)
  n18 = Round Toward -Infinity(1:w30) -> (0:w20:dbl)
  "Sample per Channel AI" <- w20
  n19 = call-poly <vilib>:"DAQmx Timing.vi"("task/channels in"=w69, "sample mode"=w51, "samples per channel"=w20, "rate"="Sample Rate", "source"="Sample Clock Source 2", "error in"=w70) -> ("task out"=w72:refnum<k21>, "error out"=w71:errorcluster)  [unwired: 8 in]
  n20 = Unbundle By Name(w2) -> ("Frequency"=w21:dbl)
  n21 = property class="DAQmx Timing"(reference=w72, error in=w71) -> (reference out=w68:refnum<k21>, error out=w67:errorcluster, "SampClk.Rate"=→"Actual Sample Rate":dbl)
  n22 = call-poly <vilib>:"DAQmx Configure Logging.vi"("task/channels in"=w68, "operation"=w66, "file path"="TDMS File Path", "logging mode"="Logging Mode", "error in"=w67) -> ("task out"=w65:refnum<k21>, "error out"=w64:errorcluster)  [unwired: 9 in]
  n23 = call-poly "VISA Configure Serial Port"("VISA resource name"="COM Port", "baud rate (9600)"="Baud Rate", "data bits (8)"="Data bits", "parity (0:none)"="Parity", "stop bits (10: 1 bit)"="stop bits") -> ("VISA resource name out"=w120:refnum<visa-resource-name>, "error out"=w126:errorcluster)  [unwired: 9 in]
  n24 = local read "Pulse generator"() -> (w1:T1)
  n25 = local write "Scan"(FALSE ("Scan")) -> ()
  n26 = call-poly <vilib>:"DAQmx Trigger.vi"("task/channels in"=w65, "source"="Pulser Trigger Source", "edge"="Edge", "error in"=w64) -> ("task out"=w48:refnum<k21>, "error out"=w47:errorcluster)  [unwired: 10 in]
  n27 = VISA Set I/O Buffer Size(VISA resource name=w120, mask (16)=48, size (4096)=u32 8192, error in (no error)=w126) -> (VISA resource name out=w116:refnum<visa-resource-name>, error out=w117:errorcluster)
  n28 = property class="DAQmx Trigger"(reference=w48, error in=w47, "Start.Retriggerable"=TRUE) -> (reference out=w29:refnum<k21>, error out=w73:errorcluster)
  n29 = local read "Y-length"() -> (w35:dbl)
  n30 = local read "Step Y"() -> (w36:dbl)
  n31 = local read "X-length"() -> (w38:dbl)
  n32 = local read "Step X"() -> (w37:dbl)
  n33 = call-poly <vilib>:"DAQmx Create Virtual Channel.vi"("maximum value"="Max Voltage 2", "minimum value"="Min Voltage 2", "physical channels"="Physical Channel(s)", "error in"=w73) -> ("task out"=w88:refnum<k21>, "error out"=w87:errorcluster)  [unwired: 10 in]
  n34 = Unbundle By Name(w1) -> ("Frequency"=w79:dbl)
  n35 = Quotient & Remainder(x=w35, y=w36) -> (floor(x/y)=w23:dbl)  [unwired: 1 out]
  n36 = Quotient & Remainder(x=w38, y=w37) -> (floor(x/y)=w25:dbl)  [unwired: 1 out]
  n37 = Build Array(w21, "Sample Rate", w25, w23) -> (w15:dbl[])
  n38 = TDMS Write(0:w27, 5:"Freq_Sampling_SizeX_SizeY" ("group name in (Untitled)"), 9:w15) -> (4:w26:refnum<k34>)  [unwired: 3 in, 3 out]
  n39 = call "PECT_GateConverse.vi"("Gate 2"="Gate 2", "Gate 1"="Gate 1", "Freq_Sampling_SizeX_SizeY"=w15) -> ("Length T/2"=w9:i32, "Length"=w10:i32, "Start 2"=w11:i32, "Start 1"=w12:i32)  [unwired: 5 in]
  n40 = Obtain Queue(max queue size (-1, unlimited)=10000, name (unnamed)="data DAQ", element data type=dbl[] [] ("data")) -> (queue out=w43:refnum<queue>)  [unwired: 2 in, 2 out]
  n41 = Increment(x=w23) -> (x+1=w24:dbl)
  n42 = Divide(x="Sample Rate 2", y=w79) -> (x/y=w77:dbl)
  n43 = Initialize Array(0.0 ("element"), w20) -> (w44:dbl[])
  n44 = Obtain Queue(max queue size (-1, unlimited)=10000, name (unnamed)="data Extraction", element data type=0.0) -> (queue out=w41:refnum<queue>)  [unwired: 2 in, 2 out]
  n45 = Multiply(x="Pulser Cycles", y=w77) -> (x*y=w75:dbl)
  n46 = call "Sigma_SetSpeed.vi"("VISA resource name"=w116, "Travel per Pulse (0.004mm)"="Travel per Pulse (mm)", "Min (1mm) 2"="2 Min", "Max (2mm) 2"="2 Max", "Rate (1mm) 2"="2 Rate", "error in (no error)"=w117, "Axis (1)"="W", "Min (1mm)"="1 Min", "Max (2mm)"="1  Max", "Rate (1mm)"="1 Rate") -> ("VISA resource name out"=w132:refnum<visa-resource-name>, "error out"=w133:errorcluster)  [unwired: 8 in]
  n47 = Round Toward -Infinity(1:w75) -> (0:w74:dbl)
  "Sample per Channel AO" <- w74
  n48 = call-poly <vilib>:"DAQmx Timing.vi"("task/channels in"=w88, "sample mode"=w103, "samples per channel"=w74, "rate"="Sample Rate 2", "source"="Sample Clock Source", "error in"=w87) -> ("task out"=w105:refnum<k21>, "error out"=w104:errorcluster)  [unwired: 8 in]
  n49 = case shown="\"                          Scan mode                      \", Default" "Tab Control 2" {
    tunnel: w29 -> [w187 w341]
    tunnel: [w186 w340] -> w54
    tunnel: [w185 w339] -> w53
    tunnel: w44 -> [w182 w338]
    tunnel: w73 -> [w184 w337]
    tunnel: w9 -> [w183 w336]
    tunnel: w43 -> [w181 _]
    tunnel: w41 -> [w173 _]
    tunnel: w25 -> [w158 _]
    tunnel: w24 -> [w179 _]
    tunnel: w10 -> [w166 w334]
    tunnel: w12 -> [w165 w333]
    tunnel: w11 -> [w164 w332]
    tunnel: w26 -> [w163 _]
    tunnel: "Waveform" ("group name in (Untitled)") -> [w160 _]
    frame "                          Scan mode                      ", Default {
      # "Column"
      # "Row"
      n50 = local read "3D Surface"() -> (w167:refnum<k7>)
      n51 = Initialize Array(-0.3 ("element"), w158, w179) -> (w172:dbl[][])
      n52 = Matrix Size(0:w172) -> (1:w174:i32, 2:w175:i32)
      n53 = Decrement(x=w174) -> (x-1=w178:i32)
      n54 = Decrement(x=w175) -> (x-1=w177:i32)
      n55 = call "Surface_AxesScale.vi"("Y-axis Max"=w177, "X-axis max"=w178, "3D Surface"=w167, "Auto Scale"=FALSE) -> ()  [unwired: 8 in]
      n56 = while {
        shift-right: [w206] -> _
        shift-left: 0 -> [w208]
        shift-right: [w205] -> _
        shift-left: 0 -> [w207]
        tunnel: w173 -> [w204]
        shift-right: [w196] -> _
        shift-left: w172 -> [w203]
        shift-right: [w197] -> _
        shift-left: TRUE ("Output Direction") -> [w198]
        stop <- w200 stop-if-true
        n57 = local read "Scan"() -> (w202:bool)
        n58 = case shown="True" w202 {
          tunnel: w208 -> [w221 w240]
          tunnel: w207 -> [w220 w239]
          tunnel: [w221 w238] -> w206
          tunnel: [w220 w237] -> w205
          tunnel: w204 -> [_ w236]
          tunnel: w203 -> [w215 w234]
          tunnel: [w216 w230] -> w196
          tunnel: [_ w233] -> w199
          tunnel: w198 -> [w219 w232]
          tunnel: [w219 w231] -> w197
          frame False {
            n59 = local read "Gate 1"() -> (w213:dbl)
            n60 = local read "Gate 2"() -> (w212:dbl)
            n61 = Wait Until Next ms Multiple(millisecond multiple=u32 100 ("ms 배수")) -> ()  [unwired: 1 out]
            n62 = call "TDMS_Open.vi"("Gate 2"=w212, "Gate 1"=w213, "Input 2D"=w215, "Open"="Open tdms") -> ("Output 2D"=w214:dbl[][])  [unwired: 6 in, 1 out]
            n63 = call "CSV Open.vi"("2D Array In"=w214, "Open"="Open csv") -> ("2D Array Out"=w218:dbl[][])  [unwired: 9 in]
            n64 = Or(x="Open tdms", y="Open csv") -> (x .or. y?=w209:bool)
            n65 = case shown="True" w209 {
              tunnel: w218 -> [w222 w224]
              tunnel: [w222 w224] -> w216
              frame False {
              }
              frame True {
                n66 = local read "3D Surface"() -> (w223:refnum<k7>)
                n67 = Matrix Size(0:w224) -> (1:w225:i32, 2:w226:i32)
                n68 = Decrement(x=w225) -> (x-1=w229:i32)
                n69 = Decrement(x=w226) -> (x-1=w228:i32)
                n70 = call "Surface_AxesScale.vi"("Y-axis Max"=w228, "X-axis max"=w229, "3D Surface"=w223, "Auto Scale"=FALSE) -> ()  [unwired: 8 in]
              }
            }
          }
          frame True {
            n71 = Dequeue Element(queue=w236) -> (element=w235:dbl)  [unwired: 2 in, 3 out]
            n72 = call "EletoMatr_1channel.vi"("Input Array X"=w234, "Input data"=w235, "In Row"=w240, "In Column"=w239, "Input Direction"=w232) -> ("Completed"=w233:bool, "Out Array X"=w230:dbl[][], "Out Row"=w238:i32, "Output Direction"=w231:bool, "Out Column"=w237:i32)  [unwired: 6 in]
          }
        }
        n73 = local read "Stop Scan"() -> (w201:bool)
        n74 = global write "Global_data.vi" "global 2d graph"(w196) -> ()
        n75 = Compound Arithmetic op=OR(w199, w201) -> (w200:bool)
        "No. Y" <- w207
        "No. X" <- w208
      }
      n76 = while {
        tunnel: w187 -> [w247]
        tunnel: [w246] -> w186
        tunnel: [w245] -> w185
        tunnel: w184 -> [w244]
        tunnel: w181 -> [w243]
        stop <- w242 stop-if-true
        n77 = case shown="True" "Scan" {
          tunnel: w247 -> [w249 w254]
          tunnel: [w249 w253] -> w246
          tunnel: [w248 w252] -> w245
          tunnel: w244 -> [w248 w251]
          tunnel: w243 -> [_ w250]
          frame False {
          }
          frame True {
            n78 = while {
              tunnel: w254 -> [w260]
              tunnel: [w266] -> w253
              tunnel: [w265] -> w252
              tunnel: w251 -> [w259]
              tunnel: w250 -> [w264]
              tunnel: [w261] -> _
              stop <- w262 stop-if-true
              n79 = First Call?() -> (First Call?: T/F=w256:bool)
              n80 = case shown="True" w256 {
                tunnel: w260 -> [w267 w272]
                tunnel: w259 -> [w268 w271]
                tunnel: [w267 w270] -> w258
                tunnel: [w268 w269] -> w257
                frame False {
                }
                frame True {
                  n81 = call <vilib>:"DAQmx Start Task.vi"("task/channels in"=w272, "error in"=w271) -> ("task out"=w270:refnum<k21>, "error out"=w269:errorcluster)  [unwired: 12 in]
                }
              }
              n82 = call-poly <vilib>:"DAQmx Read.vi"("task/channels in"=w258, "error in"=w257) -> ("task out"=w266:refnum<k21>, "data"=w255:dbl[], "error out"=w265:errorcluster)  [unwired: 11 in]
              n83 = Enqueue Element(queue=w264, element=w255) -> ()  [unwired: 2 in, 3 out]
              n84 = local read "Stop Scan"() -> (w261:bool)
              n85 = Unbundle By Name(w265) -> ("status"=w263:bool)
              n86 = Or(x=w263, y=w261) -> (x .or. y?=w262:bool)
            }
          }
        }
        n87 = local read "Stop Scan"() -> (w242:bool)
      }
      n88 = while {
        shift-right: [w285] -> _
        shift-left: w182 -> [w289]
        tunnel: w182 -> [w288]
        tunnel: w183 -> [w287]
        tunnel: w181 -> [w286]
        tunnel: w173 -> [w284]
        shift-right: [w281] -> _
        shift-left: 0 -> [w282]
        tunnel: w166 -> [w279]
        tunnel: w165 -> [w278]
        tunnel: w164 -> [w277]
        tunnel: w163 -> [w276]
        tunnel: [w275] -> w162
        tunnel: [w274] -> w161
        tunnel: w160 -> [w273]
        stop <- w280 stop-if-true
        n89 = local read "Scan"() -> (w283:bool)
        n90 = case shown="True" w283 {
          tunnel: w289 -> [w293 w304]
          tunnel: w288 -> [_ w310]
          tunnel: w287 -> [_ w309]
          tunnel: w286 -> [_ w308]
          tunnel: [w293 w307] -> w285
          tunnel: w284 -> [_ w306]
          tunnel: w282 -> [w292 w302]
          tunnel: [w292 w301] -> w281
          tunnel: w279 -> [_ w300]
          tunnel: w278 -> [_ w299]
          tunnel: w277 -> [_ w298]
          tunnel: w276 -> [w290 w297]
          tunnel: [w290 w296] -> w275
          tunnel: [_ w295] -> w274
          tunnel: w273 -> [_ w294]
          frame False {
            n91 = Wait Until Next ms Multiple(millisecond multiple=u32 100 ("ms 배수")) -> ()  [unwired: 1 out]
          }
          frame True {
            n92 = local read "Pulser Cycles"() -> (w303:i32)
            n93 = Increment(x=w302) -> (x+1=w301:i32)
            n94 = Dequeue Element(queue=w308) -> (element=w305:dbl[])  [unwired: 2 in, 3 out]
            n95 = Quotient & Remainder(x=w301, y=w303) -> (x-y*floor(x/y)=w311:i32)  [unwired: 1 out]
            n96 = Add(x=w305, y=w304) -> (x+y=w313:dbl[])
            n97 = Equal To 0?(x=w311) -> (x = 0?=w312:bool)
            n98 = case shown="True" w312 {
              tunnel: w303 -> [_ w330]
              tunnel: w313 -> [w315 w327]
              tunnel: [w315 w331] -> w307
              tunnel: w310 -> [_ w331]
              tunnel: w309 -> [_ w319]
              tunnel: w306 -> [_ w329]
              tunnel: w300 -> [_ w320]
              tunnel: w299 -> [_ w322]
              tunnel: w298 -> [_ w321]
              tunnel: w297 -> [w314 w328]
              tunnel: [w314 w326] -> w296
              tunnel: [_ w325] -> w295
              tunnel: w294 -> [_ w324]
              frame False {
                n99 = disable-structure shown="비활성화" {
                  frame Disabled {
                    n100 = Wait Until Next ms Multiple(millisecond multiple=u32 100 ("ms 배수")) -> ()  [unwired: 1 out]
                  }
                  frame Enabled {
                  }
                }
              }
              frame True {
                n101 = Divide(x=w327, y=w330) -> (x/y=w323:dbl[])
                n102 = local read "Offset"() -> (w318:bool)
                n103 = TDMS Write(0:w328, 5:w324, 9:w323) -> (4:w326:refnum<k34>, 15:w325:errorcluster)  [unwired: 3 in, 2 out]
                n104 = call "PECT_Feature extraction.vi"("Length T/2"=w319, "Offset"=w318, "Length"=w320, "Start 2"=w321, "Start 1"=w322, "Pulse signal in"=w323) -> ("Feature extraction out"=w317:dbl)  [unwired: 5 in]
                "Feature Extraction 2" <- w317
                n105 = Enqueue Element(queue=w329, element=w317) -> ()  [unwired: 2 in, 3 out]
              }
            }
          }
        }
        n106 = local read "Stop Scan"() -> (w280:bool)
        "No.data" <- w282
      }
      n107 = while {
        stop <- w194 stop-if-true
        n108 = global read "Global_data.vi" "global 2d graph"() -> (w189:dbl[][])
        n109 = Wait Until Next ms Multiple(millisecond multiple=u32 100 ("ms 배수")) -> ()  [unwired: 1 out]
        n110 = call <vilib>:"3D Surface.vi"("z matrix"=w189, "3D graph"="3D Surface") -> ()  [unwired: 8 in, 2 out]
        n111 = local read "3D Surface"() -> (w195:refnum<k7>)
        n112 = call "CSV Save.vi"("Array"=w189, "Save Button"="Save Scan mode") -> ()  [unwired: 9 in, 1 out]
        n113 = property class="CWGraph3D"(reference=w195, "ViewMode"="ViewMode") -> ()  [unwired: 1 in, 2 out]
        n114 = call <vilib>:"Basic Properties.vi"("3D graph"=w195, "plot style"="Plot style") -> ()  [unwired: 12 in, 2 out]
        n115 = local read "Stop Scan"() -> (w194:bool)
      }
      n116 = TDMS Close(8:w161, 11:w162) -> (0:w159:errorcluster)  [unwired: 1 out]
      n117 = call <vilib>:"Simple Error Handler.vi"("error in (no error)"=w159) -> ()  [unwired: 2 in, 7 out]
    }
    frame "                    Test mode                   " {
      n118 = while {
        tunnel: w341 -> [w348]
        tunnel: w337 -> [w347]
        tunnel: [w369] -> w339
        tunnel: [w370] -> w340
        shift-right: [w364] -> _
        shift-left: w338 -> [w365]
        tunnel: w338 -> [w363]
        shift-right: [w361] -> _
        shift-left: _ -> [w360]
        tunnel: w336 -> [w359]
        shift-right: [w358] -> _
        shift-left: _ -> [w357]
        shift-right: [w352] -> _
        shift-left: 1 ("Average") -> [w351]
        tunnel: w334 -> [w344]
        tunnel: w333 -> [w343]
        tunnel: w332 -> [w342]
        stop <- w371 stop-if-true
        n119 = First Call?() -> (First Call?: T/F=w349:bool)
        n120 = case shown="True" w349 {
          tunnel: w348 -> [w372 w377]
          tunnel: w347 -> [w373 w376]
          tunnel: [w372 w375] -> w346
          tunnel: [w373 w374] -> w345
          frame False {
          }
          frame True {
            n121 = call <vilib>:"DAQmx Start Task.vi"("task/channels in"=w377, "error in"=w376) -> ("task out"=w375:refnum<k21>, "error out"=w374:errorcluster)  [unwired: 12 in]
          }
        }
        n122 = local read "Pulser Cycles"() -> (w350:i32)
        n123 = call-poly <vilib>:"DAQmx Read.vi"("task/channels in"=w346, "timeout"=-1.0, "error in"=w345) -> ("task out"=w370:refnum<k21>, "data"=w353:waveform(dbl), "error out"=w369:errorcluster)  [unwired: 10 in]
        n124 = Unbundle By Name(w353) -> ("Y"=w356:dbl[])
        n125 = Quotient & Remainder(x=w351, y=w350) -> (x-y*floor(x/y)=w367:i32)  [unwired: 1 out]
        n126 = Equal To 0?(x=w367) -> (x = 0?=w366:bool)
        n127 = Add(x=w356, y=w365) -> (x+y=w362:dbl[])
        n128 = case shown="True" w366 {
          tunnel: w350 -> [_ w388]
          tunnel: w353 -> [_ w408]
          tunnel: w362 -> [w382 w407]
          tunnel: [w382 w406] -> w364
          tunnel: w363 -> [_ w406]
          tunnel: [w381 w402] -> w361
          tunnel: w360 -> [w381 w404]
          tunnel: w359 -> [_ w384]
          tunnel: [w380 w397] -> w358
          tunnel: w357 -> [w380 w399]
          tunnel: [w378 1 ("Average")] -> w352
          tunnel: w351 -> [w379 _]
          tunnel: w344 -> [_ w386]
          tunnel: w343 -> [_ w385]
          tunnel: w342 -> [_ w383]
          frame False {
            n129 = Increment(x=w379) -> (x+1=w378:i32)
          }
          frame True {
            n130 = Divide(x=w407, y=w388) -> (x/y=w391:dbl[])
            n131 = case shown="True" "Offset" {
              tunnel: w384 -> [_ w417]
              tunnel: w391 -> [w409 w411]
              tunnel: [w409 w410] -> w389
              frame False {
              }
              frame True {
                w413 = 2.0 ("y")
                n132 = Divide(x=w417, y=w413) -> (x/y=w418:dbl)
                n133 = Index Array(array=w411, index #2=w418) -> (element #1=w415:dbl, element #2=w416:dbl)  [unwired: 1 in]
                n134 = Add(x=w415, y=w416) -> (x+y=w414:dbl)
                n135 = Divide(x=w414, y=w413) -> (x/y=w412:dbl)
                n136 = Subtract(x=w411, y=w412) -> (x-y=w410:dbl[])
              }
            }
            n137 = Bundle By Name(cluster=w408, "Y"=w389) -> (w396:waveform(dbl))
            n138 = Array Subset(array=w389, index=w385, length=w386) -> (w395:dbl[])
            n139 = Array Subset(array=w389, index=w383, length=w386) -> (w394:dbl[])
            n140 = Subtract(x=w395, y=w394) -> (x-y=w393:dbl[])
            n141 = xnode "Spectral Measurements"("신호"=w396) -> ("PSD"=w400:cluster{"f0":dbl, "df":dbl, "magnitude":dbl[]})  [unwired: 1 in, 1 out]
            n142 = Add Array Elements(numeric array=w393) -> (sum=w401:dbl)
            n143 = Divide(x=w401, y=w386) -> (x/y=→"Feature Extraction":dbl)
            n144 = case shown="True" "2 Plots" {
              tunnel: [w422 w428] -> w405
              tunnel: w404 -> [_ w427]
              tunnel: [w421 w427] -> w402
              tunnel: w396 -> [w421 w423]
              tunnel: w400 -> [w419 w425]
              tunnel: [w420 w426] -> w398
              tunnel: w399 -> [_ w424]
              tunnel: [w419 w424] -> w397
              frame False {
                n145 = Build Array(w419, w419) -> (w420:cluster{"f0":dbl, "df":dbl, "magnitude":dbl[]}[])
                n146 = Build Array(w421, w421) -> (w422:waveform(dbl)[])
              }
              frame True {
                n147 = Build Array(w424, w425) -> (w426:cluster{"f0":dbl, "df":dbl, "magnitude":dbl[]}[])
                n148 = Build Array(w427, w423) -> (w428:waveform(dbl)[])
              }
            }
            "Power spectral density" <- w398
            "Hall sensors signal" <- w405
          }
        }
        n149 = local read "Stop Scan"() -> (w355:bool)
        n150 = Unbundle By Name(w369) -> ("status"=w368:bool)
        n151 = Or(x=w368, y=w355) -> (x .or. y?=w371:bool)
      }
    }
  }
  n152 = property class="DAQmx Timing"(reference=w105, error in=w104) -> (reference out=w92:refnum<k21>, error out=w97:errorcluster, "SampClk.Rate"=w95:dbl)
  "Actual Sample Rate 2" <- w95
  n153 = while {
    shift-right: [w440] -> _
    shift-left: w132 -> [w445]
    shift-right: [w442] -> _
    shift-left: w133 -> [w444]
    stop <- w441 stop-if-true
    n154 = event shown="[0] Timeout" {
      selector: _ -> [_ _ _ _ _ _ _ _ _ _ _]
      dyn-events: _ -> [_ _ _ _ _ _ _ _ _ _ _]
      timeout: 100 -> [_ _ _ _ _ _ _ _ _ _ _]
      tunnel: w445 -> [w450 w483 w496 w499 w514 w529 w544 w561 w573 w583 w595]
      tunnel: w444 -> [w449 w482 w493 w498 w513 w528 w543 w560 w572 w582 w594]
      tunnel: [w448 w483 w495 w501 w516 w531 w546 w558 w571 w585 w597] -> w440
      tunnel: [w447 w482 w494 w500 w515 w530 w545 w557 w570 w584 w596] -> w442
      tunnel: [_ "Stop Scan" _ _ _ _ _ _ _ _ _] -> w439
      event Timeout {
        n155 = event-data() -> ()  [unwired: 1 in, 2 out]
        n156 = local read "Scan"() -> (w446:bool)
        n157 = case shown="False" w446 {
          tunnel: w450 -> [w462 w481]
          tunnel: w449 -> [w461 w480]
          tunnel: [w460 w481] -> w448
          tunnel: [w459 w480] -> w447
          frame False {
            # "Stop at LS"
            n158 = local read "Travel per Pulse (mm)"() -> (w454:dbl)
            n159 = local read "Cur. Pos X"() -> (w452:dbl)
            n160 = local read "Cur. Pos Y"() -> (w451:dbl)
            n161 = call "Sigma_GetPos.vi"("VISA resource name"=w462, "Travel per Pulse (mm)"=w454, "Init Pos X (mm)"=w452, "Init  Pos Y (mm)"=w451, "error in (no error)"=w461) -> ("Pos X (mm)"=w457:dbl, "Pos Y (mm)"=w458:dbl, "VISA resource name out"=w455:refnum<visa-resource-name>, "State String"=w453:string, "error out"=w456:errorcluster)  [unwired: 6 in]
            n162 = local write "Cur. Pos X"(w457) -> ()
            n163 = local write "Cur. Pos Y"(w458) -> ()
            n164 = case shown="\"W\"" w453 {
              tunnel: [w464 w469 w474 w479] -> w460
              tunnel: [w463 w468 w473 w478] -> w459
              tunnel: w455 -> [w464 w466 w471 w476]
              tunnel: w456 -> [w463 w465 w470 w475]
              frame "K", Default {
              }
              frame "L" {
                n165 = call "Sigma_Stop.vi"("Axis (1)"="1", "error in (no error)"=w465, "VISA resource name"=w466) -> ("error out"=w468:errorcluster, "VISA resource name out"=w469:refnum<visa-resource-name>)  [unwired: 7 in]
              }
              frame "M" {
                n166 = call "Sigma_Stop.vi"("Axis (1)"="2", "error in (no error)"=w470, "VISA resource name"=w471) -> ("error out"=w473:errorcluster, "VISA resource name out"=w474:refnum<visa-resource-name>)  [unwired: 7 in]
              }
              frame "W" {
                n167 = call "Sigma_Stop.vi"("Axis (1)"="W", "error in (no error)"=w475, "VISA resource name"=w476) -> ("error out"=w478:errorcluster, "VISA resource name out"=w479:refnum<visa-resource-name>)  [unwired: 7 in]
              }
            }
          }
          frame True {
          }
        }
      }
      event "Stop Scan": Value Change {
        n168 = event-data() -> ()  [unwired: 1 in, 2 out]
      }
      event "Save Speed": Value Change {
        n169 = event-data() -> ()  [unwired: 1 in, 5 out]
        n170 = local read "Travel per Pulse (mm)"() -> (w485:dbl)
        n171 = local read "1  Max"() -> (w490:dbl)
        n172 = local read "1 Rate"() -> (w489:dbl)
        n173 = local read "2 Rate"() -> (w486:dbl)
        n174 = local read "2 Max"() -> (w487:dbl)
        n175 = local read "1 Min"() -> (w491:dbl)
        n176 = local read "2 Min"() -> (w488:dbl)
        n177 = call "Sigma_SetSpeed.vi"("VISA resource name"=w496, "Travel per Pulse (0.004mm)"=w485, "Min (1mm) 2"=w488, "Max (2mm) 2"=w487, "Rate (1mm) 2"=w486, "error in (no error)"=w493, "Axis (1)"="W", "Min (1mm)"=w491, "Max (2mm)"=w490, "Rate (1mm)"=w489) -> ("VISA resource name out"=w495:refnum<visa-resource-name>, "error out"=w494:errorcluster)  [unwired: 8 in]
      }
      event "Right": Value Change {
        n178 = event-data() -> ()  [unwired: 1 in, 1 out]
        n179 = case shown="True" "Right" {
          tunnel: [w503 w509] -> w501
          tunnel: [w502 w508] -> w500
          tunnel: w499 -> [w503 w511]
          tunnel: w498 -> [w502 w510]
          frame False {
          }
          frame True {
            n180 = local read "Travel per Pulse (mm)"() -> (w505:dbl)
            n181 = local read "Move Distance"() -> (w504:dbl)
            n182 = call "Sigma_MoveAbs.vi"("Direction (+)"=FALSE, "Axis (1)"=1, "error in (no error)"=w510, "Travel (1mm)"=w504, "Travel per Pulse (0.004mm)"=w505, "VISA resource name"=w511) -> ("error out"=w508:errorcluster, "VISA resource name out"=w509:refnum<visa-resource-name>)  [unwired: 4 in]
          }
        }
      }
      event "Left": Value Change {
        n183 = event-data() -> ()  [unwired: 1 in, 1 out]
        n184 = case shown="True" "Left" {
          tunnel: [w518 w525] -> w516
          tunnel: [w517 w524] -> w515
          tunnel: w514 -> [w518 w526]
          tunnel: w513 -> [w517 w523]
          frame False {
          }
          frame True {
            n185 = local read "Travel per Pulse (mm)"() -> (w520:dbl)
            n186 = local read "Move Distance"() -> (w519:dbl)
            n187 = call "Sigma_MoveAbs.vi"("Direction (+)"=TRUE, "Axis (1)"=1, "error in (no error)"=w523, "Travel (1mm)"=w519, "Travel per Pulse (0.004mm)"=w520, "VISA resource name"=w526) -> ("error out"=w524:errorcluster, "VISA resource name out"=w525:refnum<visa-resource-name>)  [unwired: 4 in]
          }
        }
      }
      event "Front": Value Change {
        n188 = event-data() -> ()  [unwired: 1 in, 1 out]
        n189 = case shown="True" "Front" {
          tunnel: [w533 w539] -> w531
          tunnel: [w532 w538] -> w530
          tunnel: w529 -> [w533 w541]
          tunnel: w528 -> [w532 w540]
          frame False {
          }
          frame True {
            n190 = local read "Travel per Pulse (mm)"() -> (w535:dbl)
            n191 = local read "Move Distance"() -> (w534:dbl)
            n192 = call "Sigma_MoveAbs.vi"("Direction (+)"=FALSE, "Axis (1)"=2, "error in (no error)"=w540, "Travel (1mm)"=w534, "Travel per Pulse (0.004mm)"=w535, "VISA resource name"=w541) -> ("error out"=w538:errorcluster, "VISA resource name out"=w539:refnum<visa-resource-name>)  [unwired: 4 in]
          }
        }
      }
      event "Back": Value Change {
        n193 = event-data() -> ()  [unwired: 1 in, 1 out]
        n194 = case shown="True" "Back" {
          tunnel: [w548 w554] -> w546
          tunnel: [w547 w553] -> w545
          tunnel: w544 -> [w548 w556]
          tunnel: w543 -> [w547 w555]
          frame False {
          }
          frame True {
            n195 = local read "Travel per Pulse (mm)"() -> (w550:dbl)
            n196 = local read "Move Distance"() -> (w549:dbl)
            n197 = call "Sigma_MoveAbs.vi"("Direction (+)"=TRUE, "Axis (1)"=2, "error in (no error)"=w555, "Travel (1mm)"=w549, "Travel per Pulse (0.004mm)"=w550, "VISA resource name"=w556) -> ("error out"=w553:errorcluster, "VISA resource name out"=w554:refnum<visa-resource-name>)  [unwired: 4 in]
          }
        }
      }
      event "Home X": Value Change {
        n198 = event-data() -> ()  [unwired: 1 in, 1 out]
        n199 = case shown="True" "Home X" {
          tunnel: [w563 w566] -> w558
          tunnel: [w562 w565] -> w557
          tunnel: w561 -> [w563 w568]
          tunnel: w560 -> [w562 w567]
          frame False {
          }
          frame True {
            n200 = call "Sigma_Home.vi"("Axis (1)"="1", "error in (no error)"=w567, "VISA resource name"=w568) -> ("error out"=w565:errorcluster, "VISA resource name out"=w566:refnum<visa-resource-name>)  [unwired: 7 in]
          }
        }
      }
      event "Home Y": Value Change {
        n201 = event-data() -> ()  [unwired: 1 in, 1 out]
        n202 = case shown="True" "Home Y" {
          tunnel: [w575 w578] -> w571
          tunnel: [w574 w577] -> w570
          tunnel: w573 -> [w575 w580]
          tunnel: w572 -> [w574 w579]
          frame False {
          }
          frame True {
            n203 = call "Sigma_Home.vi"("Axis (1)"="2", "error in (no error)"=w579, "VISA resource name"=w580) -> ("error out"=w577:errorcluster, "VISA resource name out"=w578:refnum<visa-resource-name>)  [unwired: 7 in]
          }
        }
      }
      event "Stop 3": Value Change {
        n204 = event-data() -> ()  [unwired: 1 in, 1 out]
        n205 = case shown="True" "Stop 3" {
          tunnel: [w587 w588] -> w585
          tunnel: [w586 w589] -> w584
          tunnel: w583 -> [w587 w591]
          tunnel: w582 -> [w586 w590]
          frame False {
          }
          frame True {
            n206 = call "Sigma_Stop.vi"("Axis (1)"="W", "error in (no error)"=w590, "VISA resource name"=w591) -> ("error out"=w589:errorcluster, "VISA resource name out"=w588:refnum<visa-resource-name>)  [unwired: 7 in]
          }
        }
      }
      event "Emergency Stop": Value Change {
        n207 = event-data() -> ()  [unwired: 1 in, 1 out]
        n208 = case shown="True" "Emergency Stop" {
          tunnel: [w599 w602] -> w597
          tunnel: [w598 w601] -> w596
          tunnel: w595 -> [w599 w604]
          tunnel: w594 -> [w598 w603]
          frame False {
          }
          frame True {
            n209 = call "Sigma_Stop.vi"("Axis (1)"="E", "error in (no error)"=w603, "VISA resource name"=w604) -> ("error out"=w601:errorcluster, "VISA resource name out"=w602:refnum<visa-resource-name>)  [unwired: 7 in]
          }
        }
      }
    }
    n210 = Unbundle By Name(w442) -> ("status"=w443:bool)
    n211 = Compound Arithmetic op=OR(w443, w439) -> (w441:bool)
  }
  n212 = Unbundle By Name("Pulse generator") -> ("Waveform Type"=w8:u16, "Frequency"=w7:dbl, "Amplitude"=w5:dbl)
  n213 = Bundle By Name(cluster=cluster{"Fs":dbl, "#s":dbl} {"Fs"=1000.0, "#s"=1000.0} ("sampling info"), "#s"=w74, "Fs"=w95) -> (w94:cluster{"Fs":dbl, "#s":dbl})
  n214 = while {
    shift-right: [w621] -> _
    shift-left: T2."No Scan" -> [w622]
    shift-right: [w617] -> _
    shift-left: 0.0 ("Current  Position (mm)") -> [w616]
    shift-right: [w615] -> _
    shift-left: 0.0 ("Current  Position (mm)") -> [w614]
    shift-right: [w613] -> _
    shift-left: 0.0 ("Current  Position (mm)") -> [w612]
    shift-right: [w611] -> _
    shift-left: 0.0 ("Current  Position (mm)") -> [w610]
    shift-right: [w618] -> w17
    shift-left: w132 -> [w620]
    shift-right: [w606] -> w18
    shift-left: w133 -> [w619]
    i -> [w605]
    stop <- w607 stop-if-true
    n215 = case shown="\"Move X\"" w622 {
      selector: w622 -> [w633 _ _ _ _]
      tunnel: [w634 T2."Wait to destination X" w698 T2."Wait to destinatioin Y" w748] -> w621
      tunnel: w620 -> [w628 w667 w692 w726 w739]
      tunnel: w619 -> [w627 w666 w691 w725 w738]
      tunnel: [w630 w669 w697 w716 w745] -> w618
      tunnel: [w629 w668 w696 w715 w744] -> w606
      tunnel: [w626 w674 w695 w722 w751] -> w617
      tunnel: w616 -> [w624 w674 w683 w722 w751]
      tunnel: [w632 w673 w700 w721 w750] -> w615
      tunnel: w614 -> [w623 w673 w700 w721 w750]
      tunnel: [w625 w672 w693 w720 w747] -> w613
      tunnel: w612 -> [_ w672 w693 w720 w733]
      tunnel: [w631 w671 w701 w719 w746] -> w611
      tunnel: w610 -> [_ w671 w701 w719 w746]
      frame "No Scan", Default {
        n216 = local read "Scan"() -> (w635:bool)
        n217 = case shown="True" w635 {
          tunnel: [w641 T2."Move X"] -> w634
          tunnel: w633 -> [w641 _]
          tunnel: w628 -> [w640 w647]
          tunnel: w627 -> [w639 w646]
          tunnel: [w640 w652] -> w630
          tunnel: [w639 w651] -> w629
          tunnel: [w638 w643] -> w626
          tunnel: [w637 w642] -> w625
          tunnel: w624 -> [w638 _]
          tunnel: w623 -> [w637 _]
          frame False {
            n218 = Wait (ms)(milliseconds to wait=u32 100) -> ()  [unwired: 1 out]
          }
          frame True {
            n219 = local read "Cur. Pos X"() -> (w649:dbl)
            n220 = local read "Cur. Pos Y"() -> (w650:dbl)
            n221 = local read "Travel per Pulse (mm)"() -> (w648:dbl)
            n222 = call "Sigma_GetPos.vi"("VISA resource name"=w647, "Travel per Pulse (mm)"=w648, "Init Pos X (mm)"=w649, "Init  Pos Y (mm)"=w650, "error in (no error)"=w646) -> ("Pos X (mm)"=w643:dbl, "Pos Y (mm)"=w642:dbl, "VISA resource name out"=w645:refnum<visa-resource-name>, "error out"=w644:errorcluster)  [unwired: 6 in, 1 out]
            "Start Pos. X" <- w643
            "Start. Pos.Y" <- w642
            n223 = local write "Cur. Pos X"(w643) -> ()
            n224 = local write "Cur. Pos Y"(w642) -> ()
            n225 = local read "Travel per Pulse (mm)"() -> (w655:dbl)
            n226 = local read "Step X"() -> (w656:dbl)
            n227 = local write "Direction (+)"(FALSE ("Direction (+)")) -> ()
            n228 = local write "Move X"(TRUE ("Move X")) -> ()
            n229 = call "Sigma_TriggerOut.vi"("Axis(1)"=1, "error in (no error)"=w644, "Trigger distance (mm)"=w656, "Travel per Pulse (mm)"=w655, "VISA resource name"=w645) -> ("error out"=w653:errorcluster, "VISA resource name out"=w654:refnum<visa-resource-name>)  [unwired: 5 in]
            n230 = flat-sequence {
              tunnel: [w663] -> w652
              tunnel: w654 -> [w663]
              tunnel: [w662] -> w651
              tunnel: w653 -> [w662]
              frame #0 {
                n231 = Wait (ms)(milliseconds to wait=u32 100) -> ()  [unwired: 1 out]
              }
            }
          }
        }
        n232 = local read "X-length"() -> (w632:dbl)
        n233 = local read "Step Y"() -> (w631:dbl)
      }
      frame "Move X" {
        n234 = local read "Travel per Pulse (mm)"() -> (w676:dbl)
        n235 = local read "X-length"() -> (w677:dbl)
        n236 = call "Sigma_MoveAbs.vi"("Direction (+)"="Direction (+)", "Axis (1)"=1, "error in (no error)"=w666, "Travel (1mm)"=w677, "Travel per Pulse (0.004mm)"=w676, "VISA resource name"=w667) -> ("error out"=w664:errorcluster, "VISA resource name out"=w665:refnum<visa-resource-name>)  [unwired: 4 in]
        n237 = flat-sequence {
          tunnel: [w681] -> w669
          tunnel: w665 -> [w681]
          tunnel: [w680] -> w668
          tunnel: w664 -> [w680]
          frame #0 {
            n238 = Wait (ms)(milliseconds to wait=u32 100) -> ()  [unwired: 1 out]
          }
        }
      }
      frame "Wait to destination X" {
        n239 = local read "Cur. Pos X"() -> (w688:dbl)
        n240 = local read "Cur. Pos Y"() -> (w687:dbl)
        n241 = local read "Travel per Pulse (mm)"() -> (w694:dbl)
        n242 = call "Sigma_GetPos.vi"("VISA resource name"=w692, "Travel per Pulse (mm)"=w694, "Init Pos X (mm)"=w688, "Init  Pos Y (mm)"=w687, "error in (no error)"=w691) -> ("Pos X (mm)"=w682:dbl, "Pos Y (mm)"=w686:dbl, "VISA resource name out"=w690:refnum<visa-resource-name>, "error out"=w689:errorcluster)  [unwired: 6 in, 1 out]
        "Cur. X" <- w682
        n243 = Absolute Value(x=w700) -> (abs(x)=w702:dbl)
        "move X" <- w702
        n244 = local write "Cur. Pos X"(w682) -> ()
        n245 = local write "Cur. Pos Y"(w686) -> ()
        n246 = Subtract(x=w682, y=w683) -> (x-y=w704:dbl)
        n247 = Absolute Value(x=w704) -> (abs(x)=w703:dbl)
        "delta X" <- w703
        n248 = Subtract(x=w703, y=w702) -> (x-y=w685:dbl)
        n249 = call "Convert Double Precision.vi"("Input"=w685) -> ("Output"=w684:dbl)  [unwired: 10 in]
        "Compare X" <- w684
        n250 = Greater Or Equal To 0?(x=w684) -> (x >= 0?=w699:bool)
        "x >= 0" <- w699
        n251 = case shown="False" w699 {
          tunnel: [T2."Wait to destination X" T2."Move Y"] -> w698
          tunnel: w690 -> [w707 w711]
          tunnel: w689 -> [w706 w710]
          tunnel: [w707 w711] -> w697
          tunnel: [w706 w710] -> w696
          tunnel: [w705 w712] -> w695
          tunnel: w683 -> [w705 _]
          frame False {
            n252 = disable-structure shown="비활성화" {
              frame Disabled {
                n253 = Wait (ms)(milliseconds to wait=u32 100) -> ()  [unwired: 1 out]
              }
              frame Enabled {
              }
            }
          }
          frame True {
            n254 = local read "Cur. Pos X"() -> (w712:dbl)
            n255 = local write "Move X"(FALSE ("Move X")) -> ()
          }
        }
        "Old X" <- w683
      }
      frame "Move Y" {
        n256 = local read "Travel per Pulse (mm)"() -> (w724:dbl)
        n257 = local read "Step Y"() -> (w727:dbl)
        n258 = call "Sigma_MoveAbs.vi"("Axis (1)"=2, "error in (no error)"=w725, "Travel (1mm)"=w727, "Travel per Pulse (0.004mm)"=w724, "VISA resource name"=w726) -> ("error out"=w717:errorcluster, "VISA resource name out"=w718:refnum<visa-resource-name>)  [unwired: 5 in]
        n259 = flat-sequence {
          tunnel: [w731] -> w716
          tunnel: w718 -> [w731]
          tunnel: [w730] -> w715
          tunnel: w717 -> [w730]
          frame #0 {
            n260 = Wait (ms)(milliseconds to wait=u32 100) -> ()  [unwired: 1 out]
          }
        }
      }
      frame "Wait to destinatioin Y" {
        n261 = local read "Cur. Pos X"() -> (w742:dbl)
        n262 = local read "Cur. Pos Y"() -> (w741:dbl)
        n263 = local read "Travel per Pulse (mm)"() -> (w743:dbl)
        n264 = call "Sigma_GetPos.vi"("VISA resource name"=w739, "Travel per Pulse (mm)"=w743, "Init Pos X (mm)"=w742, "Init  Pos Y (mm)"=w741, "error in (no error)"=w738) -> ("Pos X (mm)"=w740:dbl, "Pos Y (mm)"=w732:dbl, "VISA resource name out"=w737:refnum<visa-resource-name>, "error out"=w736:errorcluster)  [unwired: 6 in, 1 out]
        "Cur. Y" <- w732
        n265 = Absolute Value(x=w746) -> (abs(x)=w752:dbl)
        "move Y" <- w752
        n266 = Subtract(x=w732, y=w733) -> (x-y=w754:dbl)
        n267 = local write "Cur. Pos X"(w740) -> ()
        n268 = local write "Cur. Pos Y"(w732) -> ()
        n269 = Absolute Value(x=w754) -> (abs(x)=w753:dbl)
        "deltaY" <- w753
        n270 = Subtract(x=w753, y=w752) -> (x-y=w735:dbl)
        n271 = call "Convert Double Precision.vi"("Input"=w735) -> ("Output"=w734:dbl)  [unwired: 10 in]
        "compareY" <- w734
        n272 = Greater Or Equal To 0?(x=w734) -> (x >= 0?=w749:bool)
        "y >= 0" <- w749
        n273 = case shown="False" w749 {
          tunnel: [T2."Wait to destinatioin Y" w775] -> w748
          tunnel: w733 -> [w757 w770]
          tunnel: [w757 w767] -> w747
          tunnel: [w756 w765] -> w745
          tunnel: [w755 w764] -> w744
          tunnel: w737 -> [w756 w763]
          tunnel: w736 -> [w755 w762]
          frame False {
            n274 = disable-structure shown="비활성화" {
              frame Disabled {
                n275 = Wait (ms)(milliseconds to wait=u32 100) -> ()  [unwired: 1 out]
              }
              frame Enabled {
              }
            }
          }
          frame True {
            n276 = local read "Y-length"() -> (w771:dbl)
            n277 = local read "Cur. Pos Y"() -> (w767:dbl)
            n278 = local read "Start. Pos.Y"() -> (w766:dbl)
            n279 = Absolute Value(x=w771) -> (abs(x)=w772:dbl)
            n280 = Subtract(x=w766, y=w770) -> (x-y=w774:dbl)
            n281 = Absolute Value(x=w774) -> (abs(x)=w773:dbl)
            n282 = Subtract(x=w773, y=w772) -> (x-y=w761:dbl)
            n283 = local write "Move X"(FALSE ("Move X")) -> ()
            n284 = call "Convert Double Precision.vi"("Input"=w761) -> ("Output"=w760:dbl)  [unwired: 10 in]
            n285 = Greater Or Equal To 0?(x=w760) -> (x >= 0?=w768:bool)
            n286 = case shown="True" w768 {
              tunnel: [T2."Move X" T2."No Scan"] -> w775
              tunnel: [w777 w784] -> w765
              tunnel: [w776 w783] -> w764
              tunnel: w763 -> [w777 w782]
              tunnel: w762 -> [w776 w781]
              frame False {
                n287 = local read "Direction (+)"() -> (w779:bool)
                n288 = Not(x=w779) -> (.not. x?=w778:bool)
                n289 = local write "Direction (+)"(w778) -> ()
              }
              frame True {
                n290 = call "Sigma_TriggerOff.vi"("error in (no error)"=w781, "VISA resource name"=w782) -> ("error out"=w783:errorcluster, "VISA resource name out"=w784:refnum<visa-resource-name>)  [unwired: 8 in]
                n291 = local write "Scan"(FALSE ("Move X")) -> ()
              }
            }
          }
        }
        "Old.Y" <- w733
      }
    }
    n292 = local read "Stop Scan"() -> (w608:bool)
    n293 = Unbundle By Name(w606) -> ("status"=w609:bool)
    n294 = Compound Arithmetic op=OR(w609, w608) -> (w607:bool)
    "열거형" <- w622
    "숫자형" <- w605
  }
  n295 = call <vilib>:"Basic Function Generator.vi"("square wave duty cycle (%)"="Duty cycle %", "sampling info"=w94, "signal type"=w8, "error in (no error)"=w97, "amplitude"=w5, "frequency"=w7) -> ("error out"=w91:errorcluster, "signal out"=w93:waveform(dbl))  [unwired: 3 in, 1 out]
  "Waveform Graph 2" <- w93
  n296 = call-poly <vilib>:"DAQmx Trigger.vi"("task/channels in"=w92, "source"="Motor Trigger Source", "edge"=w89, "error in"=w91) -> ("task out"=w84:refnum<k21>, "error out"=w80:errorcluster)  [unwired: 10 in]
  n297 = property class="DAQmx Trigger"(reference=w84, error in=w80, "Start.Retriggerable"=TRUE) -> (reference out=w83:refnum<k21>, error out=w82:errorcluster)
  n298 = disable-structure shown="Enabled" {
    disable-tunnel: w93 -> [w791 w814]
    disable-tunnel: [w790 w813] -> w86
    disable-tunnel: [w789 w812] -> w85
    disable-tunnel: w83 -> [w788 w816]
    disable-tunnel: w82 -> [w787 w815]
    frame Disabled {
      n299 = while {
        tunnel: w791 -> [w802]
        shift-right: [w798] -> w790
        shift-left: w788 -> [w796]
        shift-right: [w797] -> w789
        shift-left: w787 -> [w795]
        stop <- FALSE stop-if-true
        n300 = call-poly <vilib>:"DAQmx Write.vi"("task/channels in"=w796, "data"=w802, "timeout"=-1.0, "error in"=w795) -> ("task out"=w801:refnum<k21>, "error out"=w800:errorcluster)  [unwired: 9 in, 1 out]
        n301 = call <vilib>:"DAQmx Start Task.vi"("task/channels in"=w801, "error in"=w800) -> ("task out"=w794:refnum<k21>, "error out"=w793:errorcluster)  [unwired: 12 in]
        n302 = disable-structure shown="활성화" {
          disable-tunnel: [w808 w810] -> w798
          disable-tunnel: [w807 w809] -> w797
          disable-tunnel: w794 -> [w806 w810]
          disable-tunnel: w793 -> [w805 w809]
          frame Disabled {
            n303 = call <vilib>:"DAQmx Wait Until Done.vi"("task/channels in"=w806, "error in"=w805) -> ("task out"=w804:refnum<k21>, "error out"=w803:errorcluster)  [unwired: 12 in]
            n304 = call <vilib>:"DAQmx Stop Task.vi"("task/channels in"=w804, "error in"=w803) -> ("task out"=w808:refnum<k21>, "error out"=w807:errorcluster)  [unwired: 12 in]
          }
          frame Enabled {
          }
        }
      }
    }
    frame Enabled {
      n305 = call-poly <vilib>:"DAQmx Write.vi"("task/channels in"=w816, "data"=w814, "timeout"=-1.0, "error in"=w815) -> ("task out"=w818:refnum<k21>, "error out"=w820:errorcluster)  [unwired: 9 in, 1 out]
      n306 = call <vilib>:"DAQmx Start Task.vi"("task/channels in"=w818, "error in"=w820) -> ("task out"=w817:refnum<k21>, "error out"=w819:errorcluster)  [unwired: 12 in]
      n307 = while {
        tunnel: w817 -> [w828]
        tunnel: w819 -> [w827]
        tunnel: [w825] -> w812
        tunnel: [w826] -> w813
        stop <- w821 stop-if-true
        n308 = call <vilib>:"DAQmx Is Task Done.vi"("task/channels in"=w828, "error in"=w827) -> ("task out"=w826:refnum<k21>, "error out"=w825:errorcluster)  [unwired: 11 in, 1 out]
        n309 = Unbundle By Name(w825) -> ("status"=w822:bool)
        n310 = Wait Until Next ms Multiple(millisecond multiple=u32 100) -> ()  [unwired: 1 out]
        n311 = Compound Arithmetic op=OR(w822, "Stop 4") -> (w821:bool)
      }
    }
  }
  n312 = call <vilib>:"DAQmx Clear Task.vi"("task in"=w86, "error in"=w85) -> ("error out"=w102:errorcluster)  [unwired: 13 in]
  n313 = VISA Close(VISA resource name=w17, error in (no error)=w18) -> (error out=w16:errorcluster)
  n314 = call <vilib>:"Simple Error Handler.vi"("error in (no error)"=w16) -> ()  [unwired: 4 in, 5 out]
  n315 = call <vilib>:"Simple Error Handler.vi"("error in (no error)"=w102) -> ()  [unwired: 4 in, 5 out]
  n316 = call <vilib>:"DAQmx Clear Task.vi"("task in"=w54, "error in"=w53) -> ("error out"=w63:errorcluster)  [unwired: 13 in]
  n317 = call <vilib>:"Simple Error Handler.vi"("error in (no error)"=w63) -> ()  [unwired: 4 in, 5 out]
  n318 = call <vilib>:"Simple Error Handler.vi"() -> ()  [unwired: 5 in, 5 out]
  "Move X" <- FALSE ("Move X")
